vi "ALONE_3AXIS_V_AMI_DESIM.vi"(6 "Refresco(s)":dbl=1.0, 8 "error in (no error)":errorcluster) -> (0 "Error Out":errorcluster, 7 "Enable":bool=TRUE)   [LabVIEW 2017]
uses:
  cRIO_ZNB_AMI_GLOBALES.vi
  AMI MAGNET/AMI 430_Hardware_Module.ctl
  AMI MAGNET/commsControl.ctl
  AMI MAGNET/magneticField.ctl
  AMI MAGNET/Status AMI.ctl
  ALONE_3AXIS_AMI.ctl
panel:
  in  "rampingMode Z 2":u16(ring)=1 items=["RAMP", "PAUSE", "MANUAL UP", "MANUAL DOWN", "ZERO"]
  in  "x":dbl min=-0.5 max=0.5 step=0.001 format="%.2f"
  in  "y":dbl min=-0.5 max=0.5 step=0.001 format="%.2f"
  in  "Vector":bool
  in  "Demag X":bool
  out "Remote DEMAG Z":bool
  out "Remote DEMAG X":bool
  out "Remote DEMAG Y":bool
  in  "Demag Y":bool
  in  "Demag Z":bool
  out "String":string="Estado"
  out "Command":T1
  out "Remote RAMP Z":bool
  out "Remote SET X":bool
  out "Remote SET Y":bool
  out "Remote RAMP X":bool
  out "Remote RAMP Y":bool
  out "Remote SET Z":bool
  in  "rampingMode X":u16(ring)=1 items=["RAMP", "PAUSE", "MANUAL UP", "MANUAL DOWN", "ZERO"]
  in  "rampingMode Y":u16(ring)=1 items=["RAMP", "PAUSE", "MANUAL UP", "MANUAL DOWN", "ZERO"]
  in  "rampingMode Z":u16(ring)=1 items=["RAMP", "PAUSE", "MANUAL UP", "MANUAL DOWN", "ZERO"]
  in  "RAMP Z":bool
  in  "SET X":bool
  out "X ramping":bool caption="Stable"
  out "X state":T2=1 items=["Unknown", "RAMPING to target field/current", "HOLDING at the target field/current", "PAUSED", "Ramping in MANUAL UP mode", "Ramping in MANUAL DOWN mode", "ZEROING CURRENT (in progress)", "Quench detected", "At ZERO current", "Heating persistent switch", "Cooling persistent switch", "External Rampdown active"]
  in  "Target X(T)":dbl min=-0.5 max=0.5 step=0.001 format="%.2f"
  in  "Rate X(T/min)":dbl=0.1 min=0.0 max=0.1 step=0.001 format="%.2f"
  out "X field (T)":dbl format="%.2f"
  in  "SET Y":bool
  out "Y ramping":bool caption="Stable"
  out "Y state":T2=1 items=["Unknown", "RAMPING to target field/current", "HOLDING at the target field/current", "PAUSED", "Ramping in MANUAL UP mode", "Ramping in MANUAL DOWN mode", "ZEROING CURRENT (in progress)", "Quench detected", "At ZERO current", "Heating persistent switch", "Cooling persistent switch", "External Rampdown active"]
  in  "Target Y(T)":dbl min=-0.5 max=0.5 step=0.001 format="%.2f"
  in  "Rate Y(T/min)":dbl=0.1 min=0.0 max=0.1 step=0.001 format="%.2f"
  out "Y field (T)":dbl format="%.2f"
  in  "RAMP X":bool
  in  "RAMP Y":bool
  in  "Settings Z":T3={"magneticFieldUnits"=1, "rampRateUnits"=1, "rampRate"=0.0, "targetField"=0.0, "rampingMode"=1} {"rampingMode" items=["RAMP", "PAUSE", "MANUAL UP", "MANUAL DOWN", "ZERO"]; "targetField" format="%.3f"; "rampRate" format="%.3f"; "rampRateUnits" items=["Per SECOND", "Per MINUTE"]; "magneticFieldUnits" items=["KGauss", "Tesla"]}
  in  "Settings Y":T3={"magneticFieldUnits"=1, "rampRateUnits"=1, "rampRate"=0.0, "targetField"=0.0, "rampingMode"=1} {"rampingMode" items=["RAMP", "PAUSE", "MANUAL UP", "MANUAL DOWN", "ZERO"]; "targetField" format="%.3f"; "rampRate" format="%.3f"; "rampRateUnits" items=["Per SECOND", "Per MINUTE"]; "magneticFieldUnits" items=["KGauss", "Tesla"]}
  in  "Settings X":T3={"magneticFieldUnits"=1, "rampRateUnits"=1, "rampRate"=0.0, "targetField"=0.0, "rampingMode"=1} {"rampingMode" items=["RAMP", "PAUSE", "MANUAL UP", "MANUAL DOWN", "ZERO"]; "targetField" format="%.3f"; "rampRate" format="%.3f"; "rampRateUnits" items=["Per SECOND", "Per MINUTE"]; "magneticFieldUnits" items=["KGauss", "Tesla"]}
  out "Waveform Chart":T4(graph)
  in  "SET Z":bool
  out "Z ramping":bool caption="Stable"
  out "Z state":T2=1 items=["Unknown", "RAMPING to target field/current", "HOLDING at the target field/current", "PAUSED", "Ramping in MANUAL UP mode", "Ramping in MANUAL DOWN mode", "ZEROING CURRENT (in progress)", "Quench detected", "At ZERO current", "Heating persistent switch", "Cooling persistent switch", "External Rampdown active"]
  out "Ciclo":i32
  in  "Target Z(T)":dbl min=-2.0 max=2.0 step=0.001 format="%.2f"
  in  "Rate Z(T/min)":dbl=0.1 min=0.0 max=0.1 step=0.001 format="%.2f"
  out "Z field (T)":dbl format="%.2f"
  out "ERROR":bool
  out "Date":string caption="asd"
  out "Time":string caption="asd"
  in  "Refresh":bool
  in  "stop":bool
  # "X axis"
  # "Z axis"
  # "STATUS"
  # "Y axis"
  # "STATUS"
  # "STATUS"
  # "SETTINGS"
  # "SETTINGS"
  # "SETTINGS"
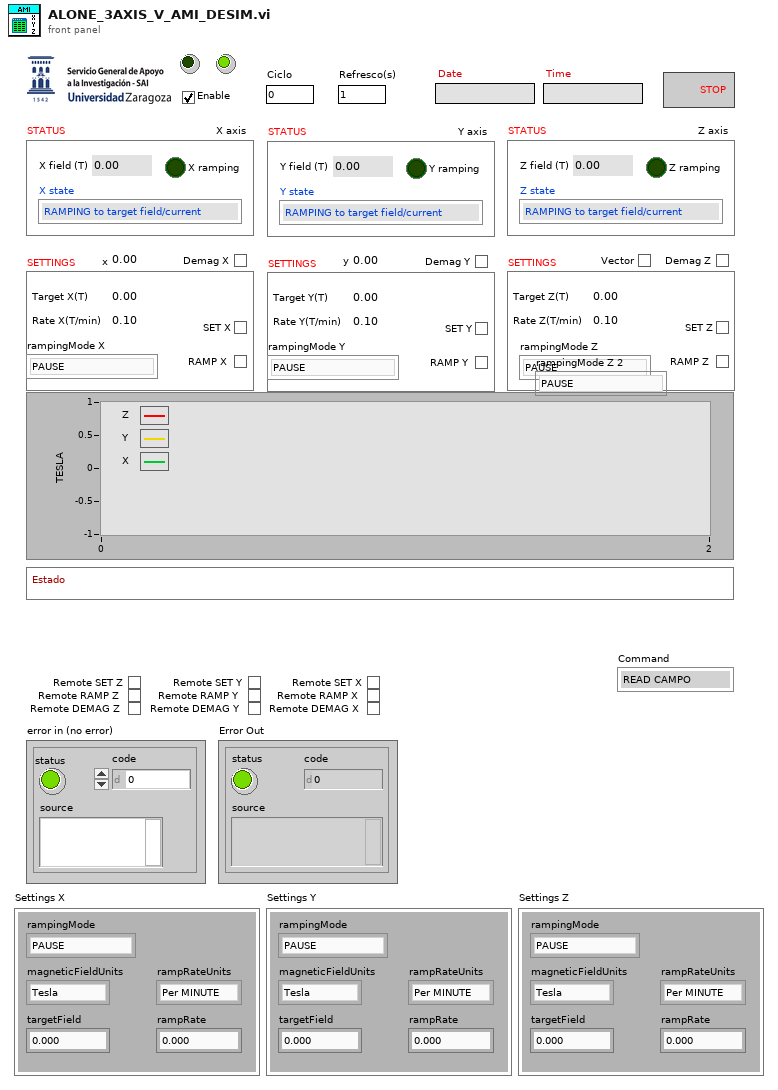
[diagram p1: front panel]
types:
  T1 = typedef "ALONE_3AXIS_AMI.ctl" = enum16{"READ CAMPO", "SET X", "SET Y", "SET Z", "RAMP X", "RAMP Y", "RAMP Z", "DESIMANAR X", "DESIMANAR Y", "DESIMANAR Z", "DESIMANAR X_RUN", "DESIMANAR Y_RUN", "DESIMANAR Z_RUN"}
  T2 = typedef "Status AMI.ctl" = u16
  T3 = typedef "magneticField.ctl" = cluster{"magneticFieldUnits":u16, "rampRateUnits":u16, "rampRate":dbl, "targetField":dbl, "rampingMode":u16}
  T4 = cluster{"magneticField":dbl, "magneticField":dbl, "magneticField":dbl}
  T5 = typedef "AMI 430_Hardware_Module.ctl" = enum16{"INICIALIZAR", "SET UNIDADES CAMPO", "SET UNIDADES RAMPA", "SET CAMPO", "SET  RAMPA", "SET RAMPING MODE", "READ CAMPO", "STATUS", "SHUTDOWN"}
  T6 = typedef "ALONE_3AXIS_AMI.ctl" = enum16{"READ CAMPO", "SET X", "SET Y", "SET Z", "RAMP X", "RAMP Y", "RAMP Z", "VECTOR Z", "DESIMANAR X", "DESIMANAR Y", "DESIMANAR Z", "DESIMANAR X_RUN", "DESIMANAR Y_RUN", "DESIMANAR Z_RUN"}
  T7 = typedef "commsControl.ctl" = cluster{"connection ID":refnum<k5>, "IP":string, "Active Comm Interface":u16, "Serial Port":refnum<visa-resource-name>, "Programmer Type":u16, "connection ID":refnum<k5>, "output cluster":cluster{"GPIB address":i16, "GPIB bus":i16}}
  T8 = cluster{"Z field (T)":dbl, "Y field (T)":dbl, "magneticField":dbl}
  T9 = cluster{"Z field (T)":dbl, "magneticField":dbl, "X field (T)":dbl}
  T10 = cluster{"magneticField":dbl, "Y field (T)":dbl, "X field (T)":dbl}
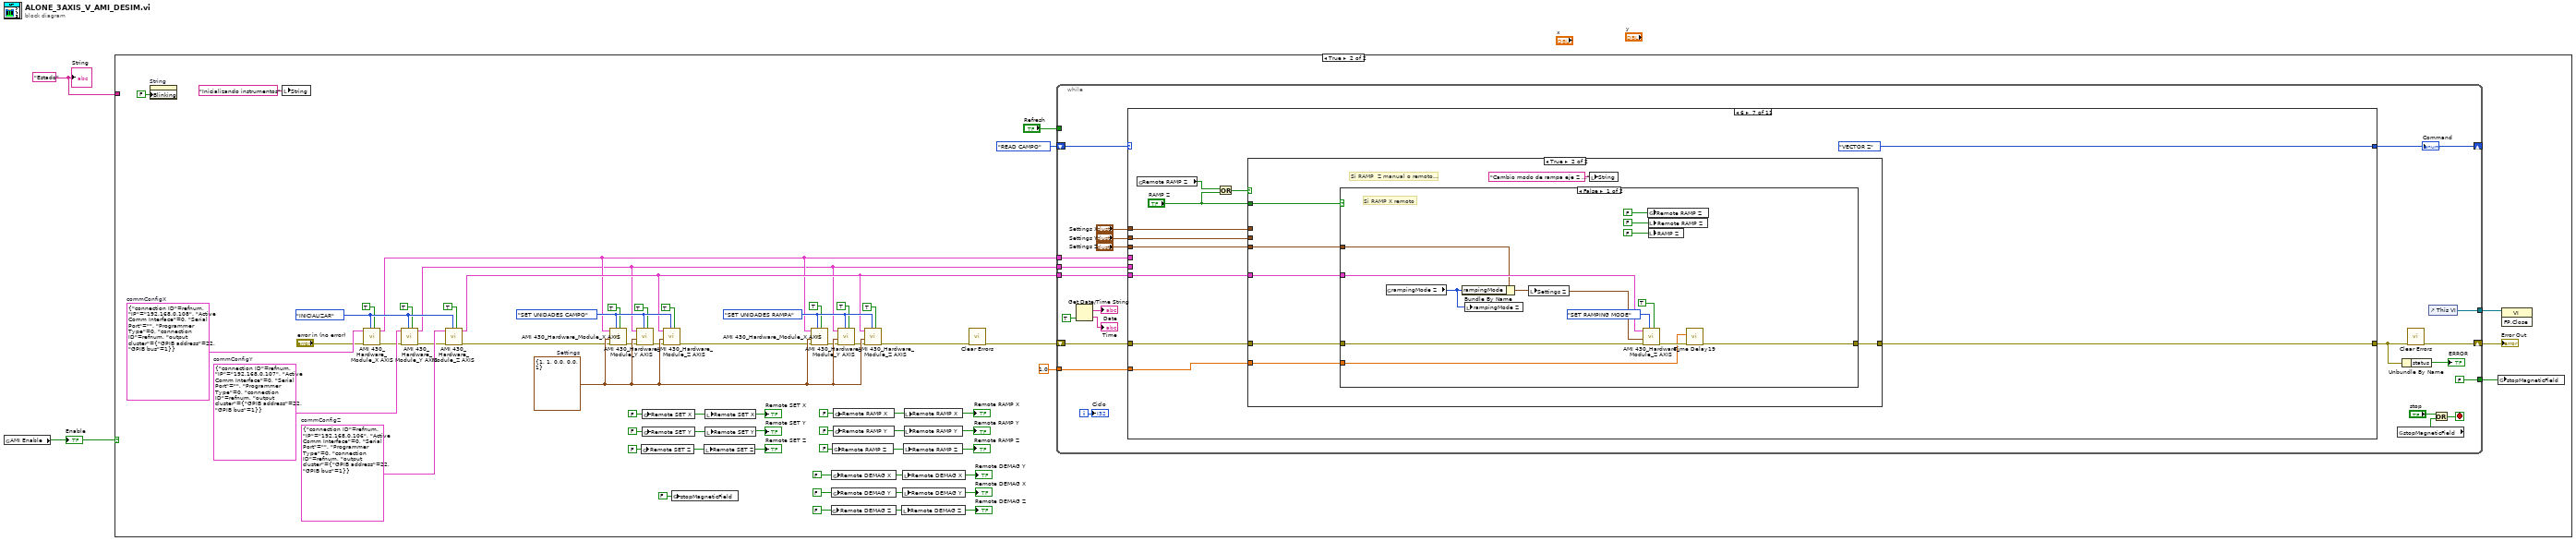
[diagram p0: block diagram]
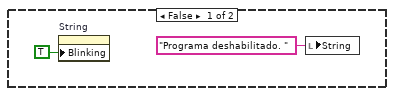
[diagram p2: hidden frame]
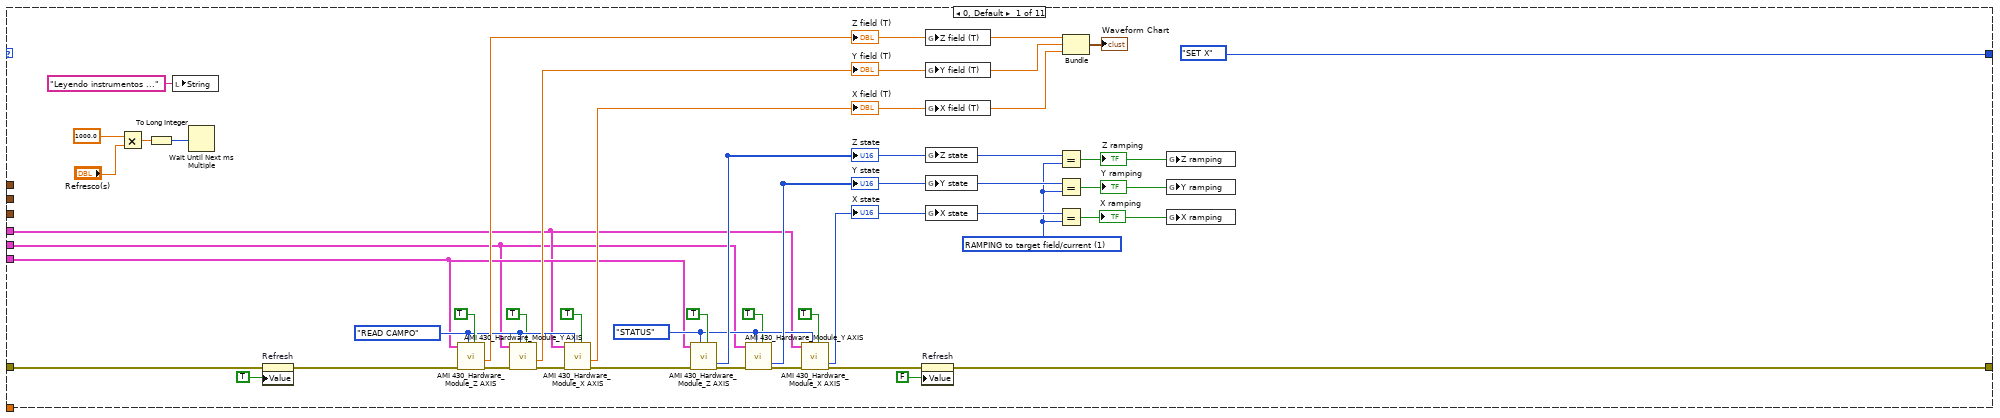
[diagram p3: hidden frame]
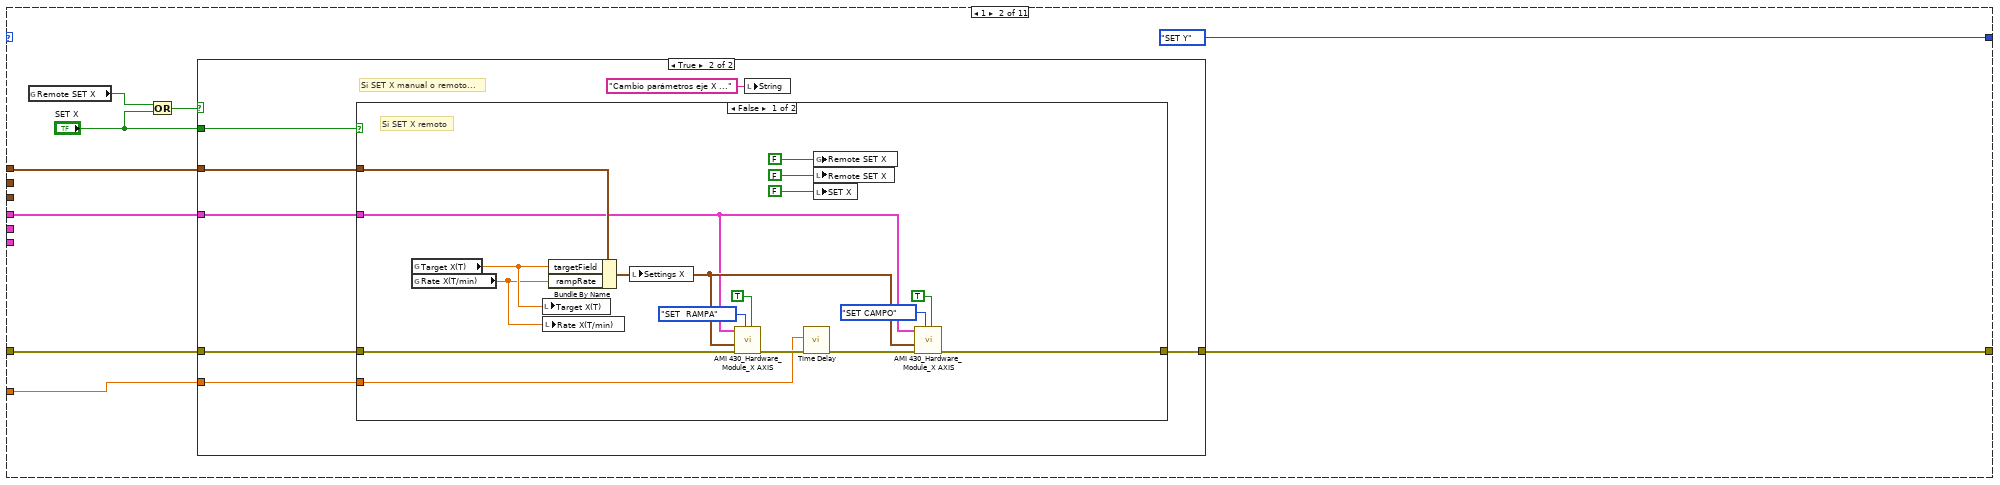
[diagram p4: hidden frame]
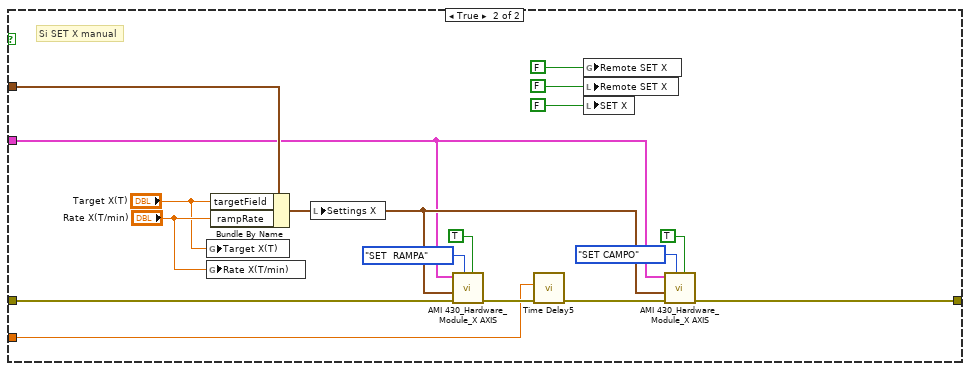
[diagram p6: hidden frame]
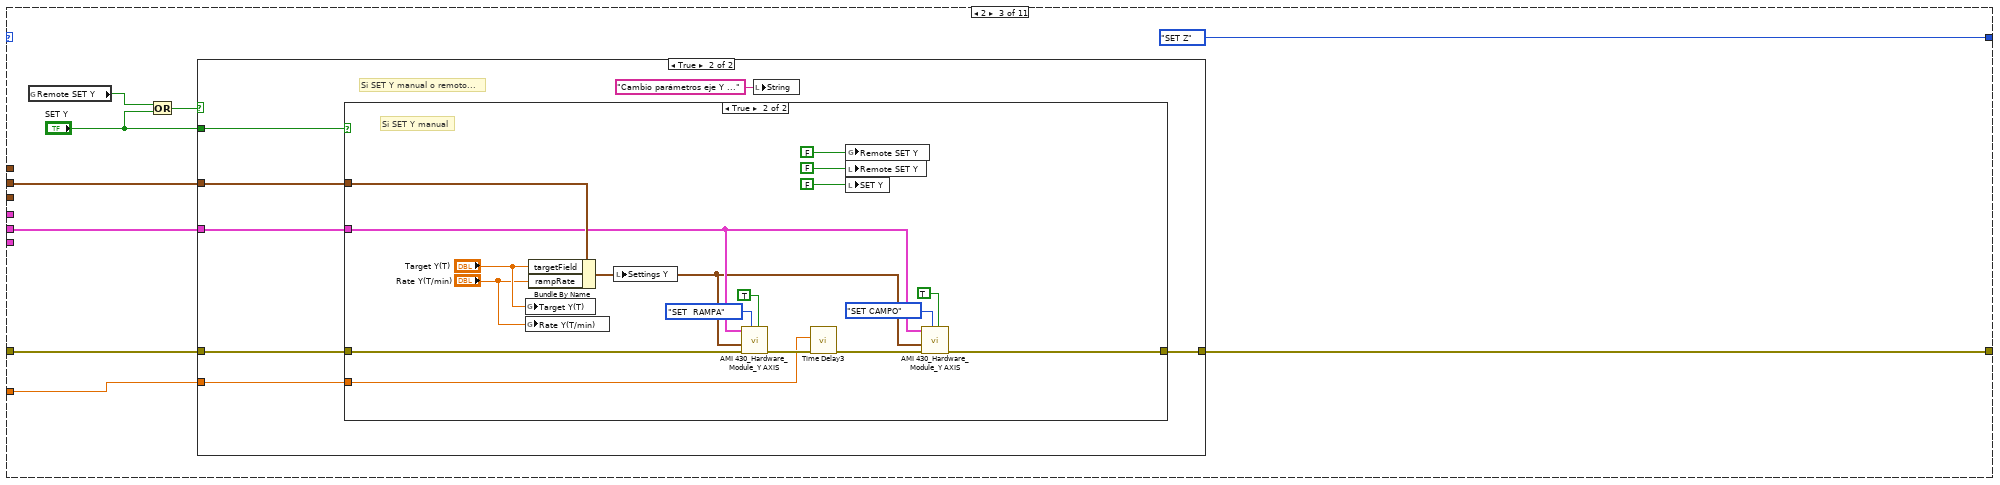
[diagram p7: hidden frame]
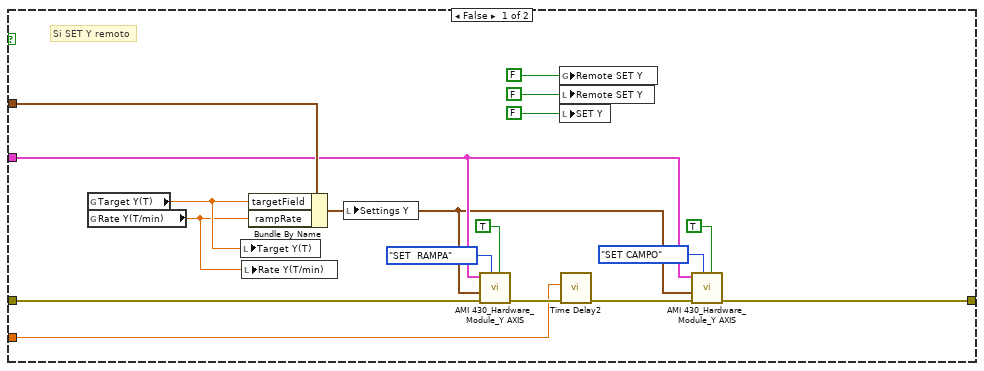
[diagram p9: hidden frame]
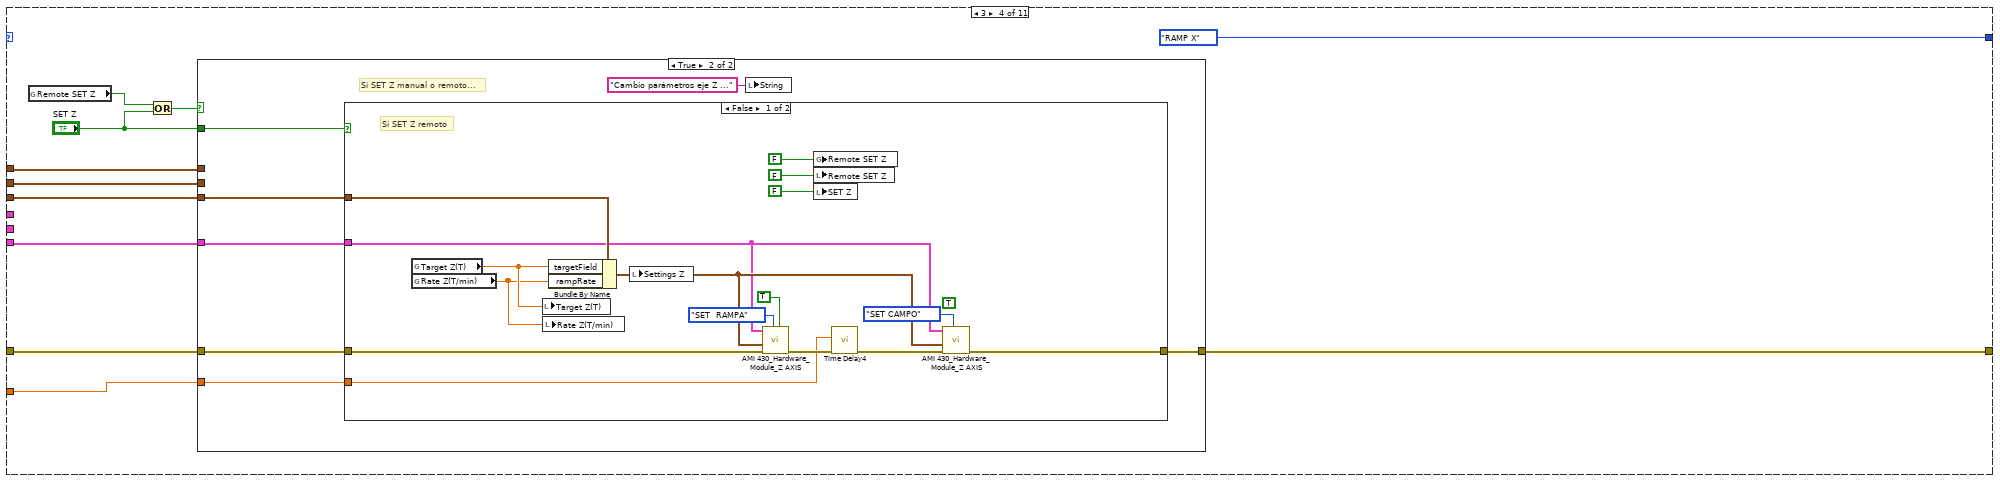
[diagram p10: hidden frame]
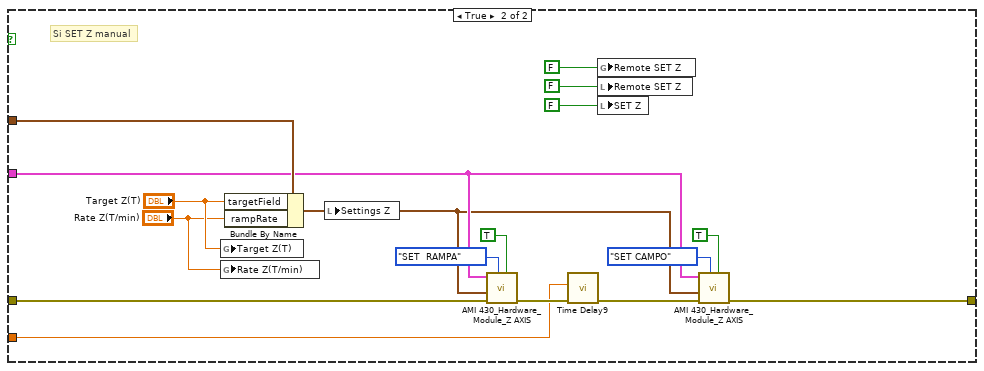
[diagram p12: hidden frame]
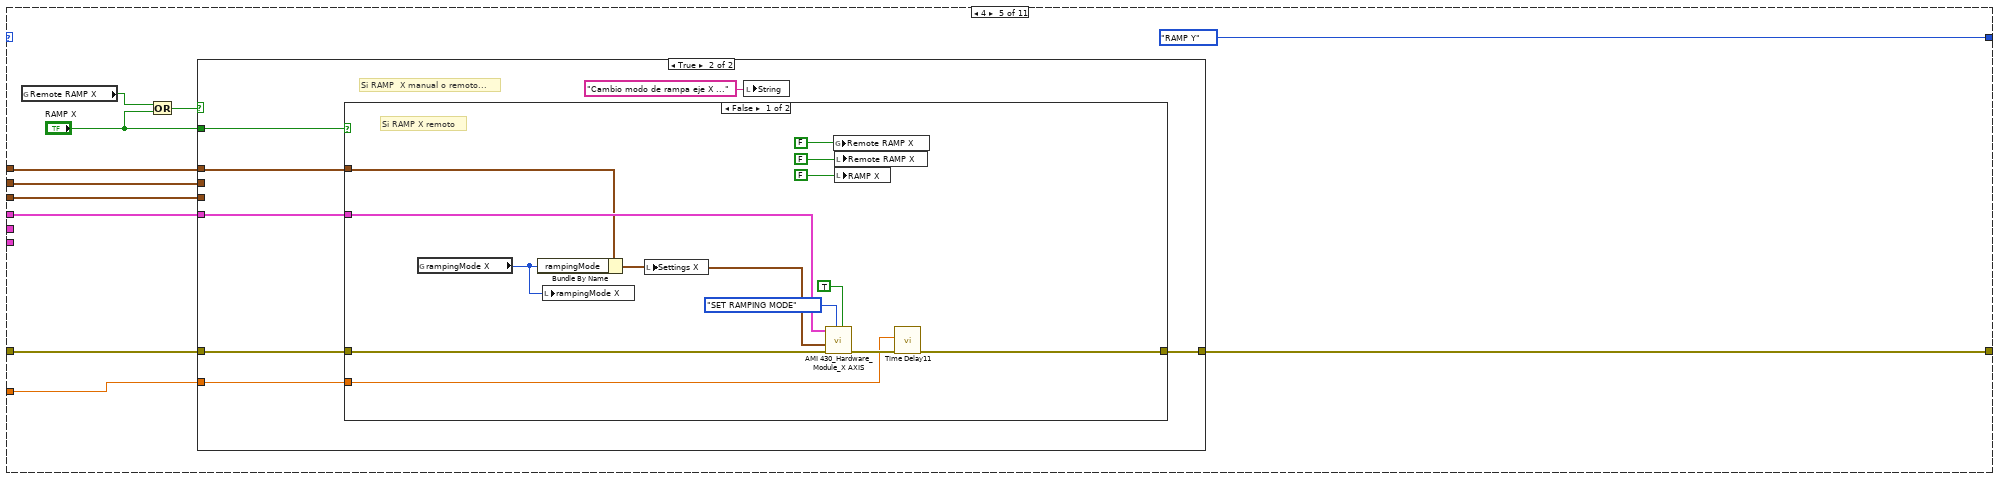
[diagram p13: hidden frame]
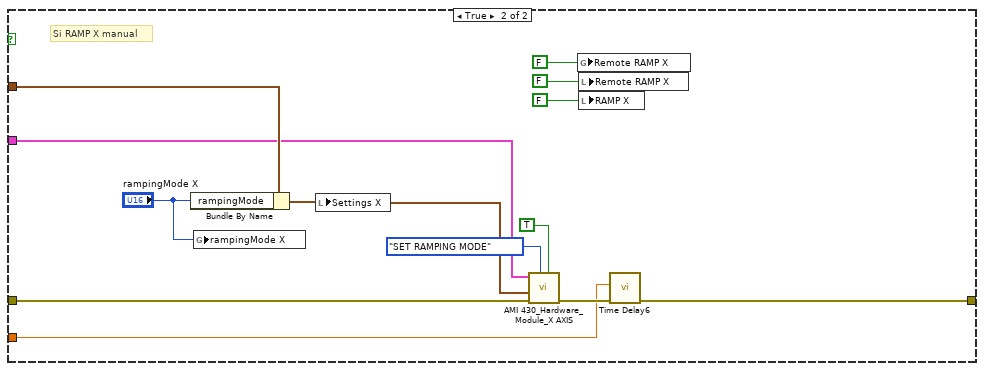
[diagram p15: hidden frame]
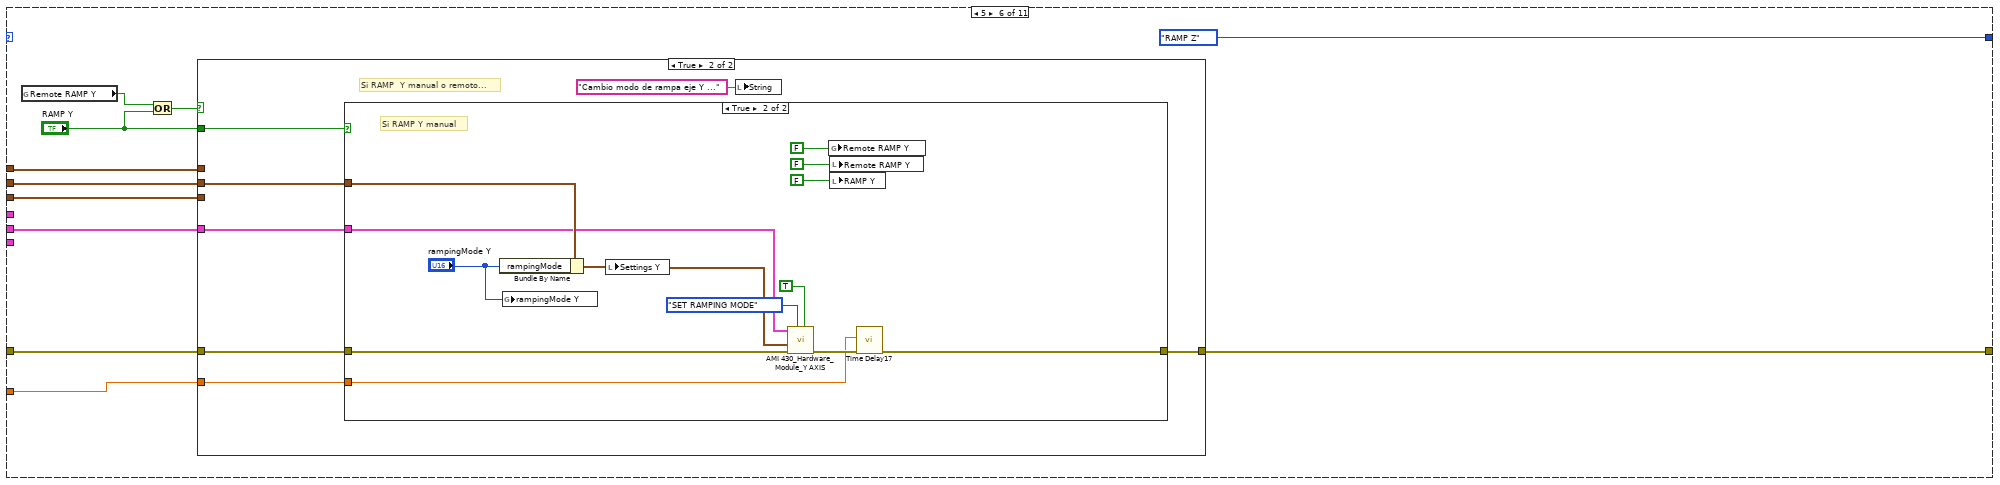
[diagram p16: hidden frame]
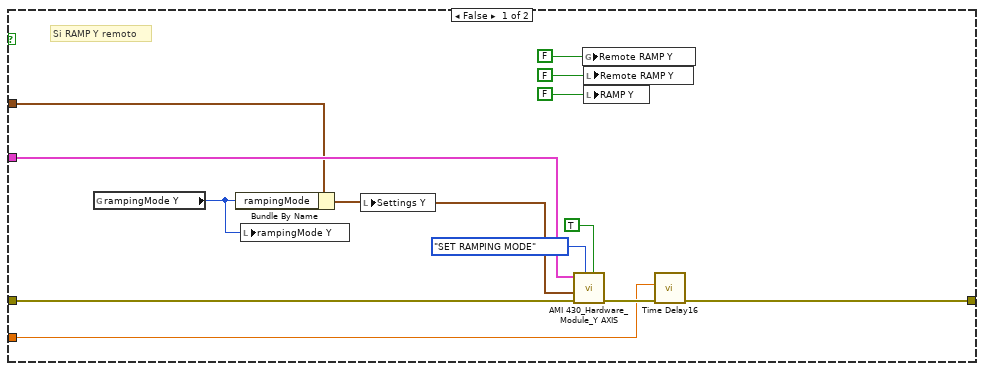
[diagram p18: hidden frame]
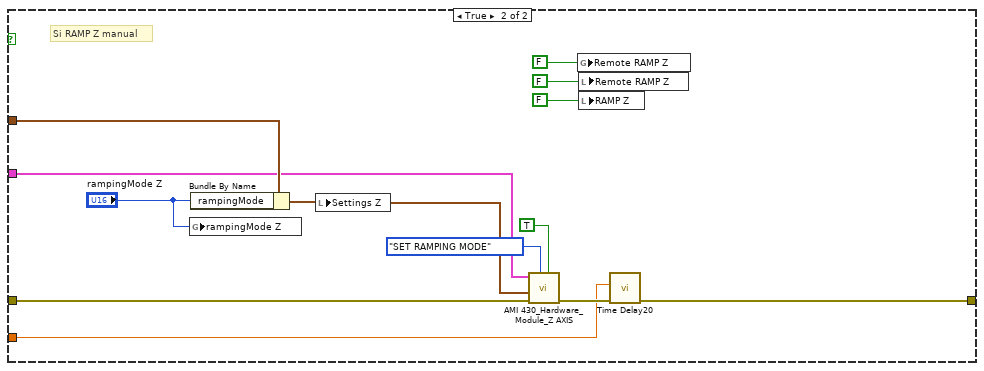
[diagram p20: hidden frame]
diagram:
  w1 = "Estado" ("String")
  n1 = global read "cRIO_ZNB_AMI_GLOBALES.vi" "AMI Enable"() -> (w2:bool)
  "Enable" <- w2
  n2 = case shown="True" w2 {
    tunnel: w1 -> [_ _]
    frame False {
      n3 = property on="String" class="Str"("Blinking"=TRUE) -> ()  [unwired: 2 in, 2 out]
      n4 = local write "String"("Programa deshabilitado. " ("String")) -> ()
    }
    frame True {
      w5 = FALSE ("Remote RAMP Z")
      w6 = FALSE ("Remote RAMP Y")
      w7 = FALSE ("Remote RAMP X")
      w12 = FALSE ("Remote SET Z")
      w11 = FALSE ("Remote SET Y")
      w13 = FALSE ("Remote SET X")
      w16 = FALSE ("Remote RAMP Z")
      w15 = FALSE ("Remote RAMP Y")
      w14 = FALSE ("Remote RAMP X")
      w45 = T3 {"magneticFieldUnits"=1, "rampRateUnits"=1, "rampRate"=0.0, "targetField"=0.0, "rampingMode"=1}  # Settings
      w41 = AMI_430_Hardware_Module."SET UNIDADES RAMPA" ("Command")
      w40 = AMI_430_Hardware_Module."SET UNIDADES CAMPO" ("Command")
      w48 = T7 {"connection ID"=refnum, "IP"="192.168.0.106", "Active Comm Interface"=0, "Serial Port"="", "Programmer Type"=0, "connection ID"=refnum, "output cluster"={"GPIB address"=22, "GPIB bus"=1}}  # commConfigZ
      w47 = T7 {"connection ID"=refnum, "IP"="192.168.0.107", "Active Comm Interface"=0, "Serial Port"="", "Programmer Type"=0, "connection ID"=refnum, "output cluster"={"GPIB address"=22, "GPIB bus"=1}}  # commConfigY
      w46 = T7 {"connection ID"=refnum, "IP"="192.168.0.108", "Active Comm Interface"=0, "Serial Port"="", "Programmer Type"=0, "connection ID"=refnum, "output cluster"={"GPIB address"=22, "GPIB bus"=1}}  # commConfigX
      w49 = AMI_430_Hardware_Module."INICIALIZAR" ("Command")
      n5 = property on="String" class="Str"("Blinking"=FALSE) -> ()  [unwired: 2 in, 2 out]
      n6 = local write "String"("Inicializando instrumentos" ("String")) -> ()
      n7 = call "AMI 430_Hardware_Module_X AXIS.vi"("Enable"=TRUE, "Command"=w49, "error in (no error)"="error in (no error)", "Comm Config In"=w46) -> ("error out"=w36:errorcluster, "Comm Config Out"=w20:T7)  [unwired: 3 in, 3 out]
      n8 = call "AMI 430_Hardware_Module_Y AXIS.vi"("Enable"=TRUE, "Command"=w49, "error in (no error)"=w36, "Comm Config In"=w47) -> ("error out"=w35:errorcluster, "Comm Config Out"=w19:T7)  [unwired: 3 in, 3 out]
      n9 = call "AMI 430_Hardware_Module_Z AXIS.vi"("Enable"=TRUE, "Command"=w49, "error in (no error)"=w35, "Comm Config In"=w48) -> ("error out"=w39:errorcluster, "Comm Config Out"=w21:T7)  [unwired: 3 in, 3 out]
      n10 = call "AMI 430_Hardware_Module_X AXIS.vi"("Enable"=TRUE, "Command"=w40, "error in (no error)"=w39, "Settings"=w45, "Comm Config In"=w20) -> ("error out"=w37:errorcluster)  [unwired: 2 in, 4 out]
      n11 = call "AMI 430_Hardware_Module_Y AXIS.vi"("Enable"=TRUE, "Command"=w40, "error in (no error)"=w37, "Settings"=w45, "Comm Config In"=w19) -> ("error out"=w38:errorcluster)  [unwired: 2 in, 4 out]
      n12 = global write "cRIO_ZNB_AMI_GLOBALES.vi" "Remote SET Z"(w12) -> ()
      n13 = global write "cRIO_ZNB_AMI_GLOBALES.vi" "Remote SET X"(w13) -> ()
      n14 = global write "cRIO_ZNB_AMI_GLOBALES.vi" "Remote SET Y"(w11) -> ()
      n15 = call "AMI 430_Hardware_Module_Z AXIS.vi"("Enable"=TRUE, "Command"=w40, "error in (no error)"=w38, "Settings"=w45, "Comm Config In"=w21) -> ("error out"=w44:errorcluster)  [unwired: 2 in, 4 out]
      n16 = global write "cRIO_ZNB_AMI_GLOBALES.vi" "stopMagneticField"(FALSE ("stopMagneticField")) -> ()
      n17 = local write "Remote SET Z"(w12) -> ()
      n18 = local write "Remote SET X"(w13) -> ()
      n19 = local write "Remote SET Y"(w11) -> ()
      n20 = call "AMI 430_Hardware_Module_X AXIS.vi"("Enable"=TRUE, "Command"=w41, "error in (no error)"=w44, "Settings"=w45, "Comm Config In"=w20) -> ("error out"=w42:errorcluster)  [unwired: 2 in, 4 out]
      n21 = global write "cRIO_ZNB_AMI_GLOBALES.vi" "Remote DEMAG Z"(w5) -> ()
      n22 = global write "cRIO_ZNB_AMI_GLOBALES.vi" "Remote DEMAG X"(w7) -> ()
      n23 = global write "cRIO_ZNB_AMI_GLOBALES.vi" "Remote DEMAG Y"(w6) -> ()
      n24 = global write "cRIO_ZNB_AMI_GLOBALES.vi" "Remote RAMP Z"(w16) -> ()
      n25 = global write "cRIO_ZNB_AMI_GLOBALES.vi" "Remote RAMP X"(w14) -> ()
      n26 = global write "cRIO_ZNB_AMI_GLOBALES.vi" "Remote RAMP Y"(w15) -> ()
      n27 = call "AMI 430_Hardware_Module_Y AXIS.vi"("Enable"=TRUE, "Command"=w41, "error in (no error)"=w42, "Settings"=w45, "Comm Config In"=w19) -> ("error out"=w43:errorcluster)  [unwired: 2 in, 4 out]
      n28 = call "AMI 430_Hardware_Module_Z AXIS.vi"("Enable"=TRUE, "Command"=w41, "error in (no error)"=w43, "Settings"=w45, "Comm Config In"=w21) -> ("error out"=w34:errorcluster)  [unwired: 2 in, 4 out]
      n29 = local write "Remote DEMAG Z"(w5) -> ()
      n30 = local write "Remote DEMAG X"(w7) -> ()
      n31 = local write "Remote DEMAG Y"(w6) -> ()
      n32 = local write "Remote RAMP Z"(w16) -> ()
      n33 = local write "Remote RAMP X"(w14) -> ()
      n34 = local write "Remote RAMP Y"(w15) -> ()
      n35 = call <vilib>:"Clear Errors.vi"("error in (no error)"=w34) -> ("error out"=w18:errorcluster)  [unwired: 5 in, 1 out]
      n36 = while {
        shift-right: [w65] -> w50
        shift-left: w18 -> [w58]
        tunnel: [FALSE ("stop")] -> w51
        tunnel: [w68] -> w52
        tunnel: "Refresh" -> [_]
        tunnel: w19 -> [w59]
        tunnel: w21 -> [w60]
        tunnel: w20 -> [w61]
        shift-right: [w54] -> _
        shift-left: ALONE_3AXIS_AMI."READ CAMPO" ("Command") -> [w63]
        tunnel: 1.0 ("Delay Time (s)") -> [w53]
        i -> [w64]
        stop <- w72 stop-if-true
        n37 = Get Date/Time String(want seconds? (F)=TRUE) -> (date string=→"Date":string, time string=→"Time":string)  [unwired: 2 in]
        n38 = case shown="6" w63 {
          tunnel: w58 -> [w78 w121 w173 w225 w277 w322 w367 w412 w457 w540 w624]
          tunnel: w61 -> [w88 w117 _ _ w268 _ _ _ w449 _ _]
          tunnel: w59 -> [w87 _ w165 _ _ w314 _ _ _ w531 _]
          tunnel: w60 -> [w89 _ _ w216 _ _ w358 w404 _ _ w615]
          tunnel: [w75 w120 w172 w224 w276 w321 w366 w411 w456 w539 w623] -> w62
          tunnel: "Settings Y" -> [_ _ w166 w217 w270 w315 w360 w405 w450 w533 w617]
          tunnel: "Settings Z" -> [_ _ _ w218 w271 w316 w361 w406 w451 w534 w618]
          tunnel: "Settings X" -> [_ w122 _ w226 w278 w323 w368 w413 w458 w541 w625]
          tunnel: [ALONE_3AXIS_AMI."SET X" ("Command") ALONE_3AXIS_AMI."SET Y" ("Command") ALONE_3AXIS_AMI."SET Z" ("Command") ALONE_3AXIS_AMI."RAMP X" ("Command") ALONE_3AXIS_AMI."RAMP Y" ("Command") ALONE_3AXIS_AMI."RAMP Z" ("Command") ALONE_3AXIS_AMI."VECTOR Z" ("Command") ALONE_3AXIS_AMI."DESIMANAR X" ("Command") ALONE_3AXIS_AMI."DESIMANAR Y" ("Command") ALONE_3AXIS_AMI."DESIMANAR Z" ("Command") ALONE_3AXIS_AMI."READ CAMPO" ("Command")] -> w54
          tunnel: w53 -> [_ w118 w170 w222 w274 w319 w364 w409 w454 w537 w621]
          frame 0, Default {
            w98 = T2 1 items=["Unknown", "RAMPING to target field/current", "HOLDING at the target field/current", "PAUSED", "Ramping in MANUAL UP mode", "Ramping in MANUAL DOWN mode", "ZEROING CURRENT (in progress)", "Quench detected", "At ZERO current", "Heating persistent switch", "Cooling persistent switch", "External Rampdown active"] ("y")
            w96 = AMI_430_Hardware_Module."STATUS" ("Command")
            w92 = AMI_430_Hardware_Module."READ CAMPO" ("Command")
            n39 = Multiply(x=1000.0, y="Refresco(s)") -> (x*y=w83:dbl)
            n40 = To Long Integer(number=w83) -> (32bit integer=w81:i32)
            n41 = local write "String"("Leyendo instrumentos ..." ("String")) -> ()
            n42 = Wait Until Next ms Multiple(millisecond multiple=w81) -> ()  [unwired: 1 out]
            n43 = property on="Refresh" class="Bool (strict)"(error in=w78, "Value"=TRUE ("Refresh")) -> (error out=w77:errorcluster)  [unwired: 1 in, 1 out]
            n44 = call "AMI 430_Hardware_Module_Z AXIS.vi"("Enable"=TRUE, "Command"=w92, "error in (no error)"=w77, "Comm Config In"=w89) -> ("error out"=w100:errorcluster, "magneticField"=w110:dbl)  [unwired: 3 in, 3 out]
            "Z field (T)" <- w110
            n45 = call "AMI 430_Hardware_Module_Y AXIS.vi"("Enable"=TRUE, "Command"=w92, "error in (no error)"=w100, "Comm Config In"=w87) -> ("error out"=w99:errorcluster, "magneticField"=w109:dbl)  [unwired: 3 in, 3 out]
            "Y field (T)" <- w109
            n46 = call "AMI 430_Hardware_Module_X AXIS.vi"("Enable"=TRUE, "Command"=w92, "error in (no error)"=w99, "Comm Config In"=w88) -> ("error out"=w101:errorcluster, "magneticField"=w108:dbl)  [unwired: 3 in, 3 out]
            "X field (T)" <- w108
            n47 = call "AMI 430_Hardware_Module_Z AXIS.vi"("Enable"=TRUE, "Command"=w96, "error in (no error)"=w101, "Comm Config In"=w89) -> ("error out"=w103:errorcluster, "state"=w111:T2)  [unwired: 3 in, 3 out]
            "Z state" <- w111
            n48 = call "AMI 430_Hardware_Module_Y AXIS.vi"("Enable"=TRUE, "Command"=w96, "error in (no error)"=w103, "Comm Config In"=w87) -> ("error out"=w102:errorcluster, "state"=w112:T2)  [unwired: 3 in, 3 out]
            "Y state" <- w112
            n49 = call "AMI 430_Hardware_Module_X AXIS.vi"("Enable"=TRUE, "Command"=w96, "error in (no error)"=w102, "Comm Config In"=w88) -> ("error out"=w76:errorcluster, "state"=w113:T2)  [unwired: 3 in, 3 out]
            "X state" <- w113
            n50 = property on="Refresh" class="Bool (strict)"(error in=w76, "Value"=FALSE ("Refresh")) -> (error out=w75:errorcluster)  [unwired: 1 in, 1 out]
            n51 = global write "cRIO_ZNB_AMI_GLOBALES.vi" "Z field (T)"(w110) -> ()
            n52 = global write "cRIO_ZNB_AMI_GLOBALES.vi" "Y field (T)"(w109) -> ()
            n53 = global write "cRIO_ZNB_AMI_GLOBALES.vi" "X field (T)"(w108) -> ()
            n54 = global write "cRIO_ZNB_AMI_GLOBALES.vi" "Z state"(w111) -> ()
            n55 = global write "cRIO_ZNB_AMI_GLOBALES.vi" "Y state"(w112) -> ()
            n56 = global write "cRIO_ZNB_AMI_GLOBALES.vi" "X state"(w113) -> ()
            n57 = Equal?(x=w111, y=w98) -> (x = y?=w105:bool)
            "Z ramping" <- w105
            n58 = Equal?(x=w112, y=w98) -> (x = y?=w107:bool)
            "Y ramping" <- w107
            n59 = Equal?(x=w113, y=w98) -> (x = y?=w106:bool)
            "X ramping" <- w106
            n60 = Bundle("magneticField"=w110, "magneticField"=w109, "magneticField"=w108) -> (→"Waveform Chart":T4)  [unwired: 1 in]
            n61 = global write "cRIO_ZNB_AMI_GLOBALES.vi" "Z ramping"(w105) -> ()
            n62 = global write "cRIO_ZNB_AMI_GLOBALES.vi" "Y ramping"(w107) -> ()
            n63 = global write "cRIO_ZNB_AMI_GLOBALES.vi" "X ramping"(w106) -> ()
          }
          frame 1 {
            n64 = global read "cRIO_ZNB_AMI_GLOBALES.vi" "Remote SET X"() -> (w116:bool)
            n65 = Or(x=w116, y="SET X") -> (x .or. y?=w115:bool)
            n66 = case shown="True" w115 {
              tunnel: w122 -> [_ w130]
              tunnel: w121 -> [w123 w129]
              tunnel: [w123 w128] -> w120
              tunnel: w118 -> [_ w127]
              tunnel: w117 -> [_ w126]
              tunnel: "SET X" -> [_ w125]
              frame False {
              }
              frame True {
                # "Si SET X manual o remoto..."
                n67 = case shown="False" w125 {
                  tunnel: w130 -> [w140 w155]
                  tunnel: w129 -> [w139 w154]
                  tunnel: [w138 w153] -> w128
                  tunnel: w127 -> [w137 w152]
                  tunnel: w126 -> [w136 w151]
                  frame False {
                    # "Si SET X remoto"
                    n68 = global read "cRIO_ZNB_AMI_GLOBALES.vi" "Target X(T)"() -> (w135:dbl)
                    n69 = global read "cRIO_ZNB_AMI_GLOBALES.vi" "Rate X(T/min)"() -> (w134:dbl)
                    n70 = local write "Target X(T)"(w135) -> ()
                    n71 = local write "Rate X(T/min)"(w134) -> ()
                    n72 = Bundle By Name(cluster=w140, "targetField"=w135, "rampRate"=w134) -> (w147:T3)
                    n73 = local write "Settings X"(w147) -> ()
                    n74 = call "AMI 430_Hardware_Module_X AXIS.vi"("Enable"=TRUE, "Command"=AMI_430_Hardware_Module."SET  RAMPA", "error in (no error)"=w139, "Settings"=w147, "Comm Config In"=w136) -> ("error out"=w145:errorcluster)  [unwired: 2 in, 4 out]
                    n75 = call "Time Delay"("error in (no error)"=w145, "Delay Time (s)"=w137) -> ("error out"=w146:errorcluster)  [unwired: 9 in]
                    n76 = global write "cRIO_ZNB_AMI_GLOBALES.vi" "Remote SET X"(FALSE ("Remote SET X")) -> ()
                    n77 = local write "Remote SET X"(FALSE ("Remote SET X")) -> ()
                    n78 = local write "SET X"(FALSE ("Remote SET X")) -> ()
                    n79 = call "AMI 430_Hardware_Module_X AXIS.vi"("Enable"=TRUE, "Command"=AMI_430_Hardware_Module."SET CAMPO", "error in (no error)"=w146, "Settings"=w147, "Comm Config In"=w136) -> ("error out"=w138:errorcluster)  [unwired: 2 in, 4 out]
                  }
                  frame True {
                    # "Si SET X manual"
                    n80 = global write "cRIO_ZNB_AMI_GLOBALES.vi" "Target X(T)"("Target X(T)") -> ()
                    n81 = global write "cRIO_ZNB_AMI_GLOBALES.vi" "Rate X(T/min)"("Rate X(T/min)") -> ()
                    n82 = Bundle By Name(cluster=w155, "targetField"="Target X(T)", "rampRate"="Rate X(T/min)") -> (w162:T3)
                    n83 = local write "Settings X"(w162) -> ()
                    n84 = call "AMI 430_Hardware_Module_X AXIS.vi"("Enable"=TRUE, "Command"=AMI_430_Hardware_Module."SET  RAMPA", "error in (no error)"=w154, "Settings"=w162, "Comm Config In"=w151) -> ("error out"=w160:errorcluster)  [unwired: 2 in, 4 out]
                    n85 = call "Time Delay5"("error in (no error)"=w160, "Delay Time (s)"=w152) -> ("error out"=w161:errorcluster)  [unwired: 9 in]
                    n86 = global write "cRIO_ZNB_AMI_GLOBALES.vi" "Remote SET X"(FALSE ("Remote SET X")) -> ()
                    n87 = local write "Remote SET X"(FALSE ("Remote SET X")) -> ()
                    n88 = local write "SET X"(FALSE ("Remote SET X")) -> ()
                    n89 = call "AMI 430_Hardware_Module_X AXIS.vi"("Enable"=TRUE, "Command"=AMI_430_Hardware_Module."SET CAMPO", "error in (no error)"=w161, "Settings"=w162, "Comm Config In"=w151) -> ("error out"=w153:errorcluster)  [unwired: 2 in, 4 out]
                  }
                }
                n90 = local write "String"("Cambio parámetros eje X ..." ("String")) -> ()
              }
            }
          }
          frame 2 {
            n91 = global read "cRIO_ZNB_AMI_GLOBALES.vi" "Remote SET Y"() -> (w169:bool)
            n92 = Or(x=w169, y="SET Y") -> (x .or. y?=w168:bool)
            n93 = case shown="True" w168 {
              tunnel: w166 -> [_ w181]
              tunnel: w173 -> [w174 w180]
              tunnel: [w174 w179] -> w172
              tunnel: w170 -> [_ w178]
              tunnel: w165 -> [_ w177]
              tunnel: "SET Y" -> [_ w176]
              frame False {
              }
              frame True {
                # "Si SET Y manual o remoto..."
                n94 = case shown="True" w176 {
                  tunnel: w181 -> [w198 w215]
                  tunnel: w180 -> [w184 w205]
                  tunnel: [w182 w204] -> w179
                  tunnel: w178 -> [w183 w203]
                  tunnel: w177 -> [w186 w202]
                  frame False {
                    # "Si SET Y remoto"
                    n95 = global read "cRIO_ZNB_AMI_GLOBALES.vi" "Target Y(T)"() -> (w197:dbl)
                    n96 = global read "cRIO_ZNB_AMI_GLOBALES.vi" "Rate Y(T/min)"() -> (w196:dbl)
                    n97 = local write "Target Y(T)"(w197) -> ()
                    n98 = local write "Rate Y(T/min)"(w196) -> ()
                    n99 = Bundle By Name(cluster=w198, "targetField"=w197, "rampRate"=w196) -> (w185:T3)
                    n100 = local write "Settings Y"(w185) -> ()
                    n101 = call "AMI 430_Hardware_Module_Y AXIS.vi"("Enable"=TRUE, "Command"=AMI_430_Hardware_Module."SET  RAMPA", "error in (no error)"=w184, "Settings"=w185, "Comm Config In"=w186) -> ("error out"=w192:errorcluster)  [unwired: 2 in, 4 out]
                    n102 = global write "cRIO_ZNB_AMI_GLOBALES.vi" "Remote SET Y"(FALSE ("Remote SET X")) -> ()
                    n103 = local write "Remote SET Y"(FALSE ("Remote SET X")) -> ()
                    n104 = local write "SET Y"(FALSE ("Remote SET X")) -> ()
                    n105 = call "Time Delay2"("error in (no error)"=w192, "Delay Time (s)"=w183) -> ("error out"=w190:errorcluster)  [unwired: 9 in]
                    n106 = call "AMI 430_Hardware_Module_Y AXIS.vi"("Enable"=TRUE, "Command"=AMI_430_Hardware_Module."SET CAMPO", "error in (no error)"=w190, "Settings"=w185, "Comm Config In"=w186) -> ("error out"=w182:errorcluster)  [unwired: 2 in, 4 out]
                  }
                  frame True {
                    # "Si SET Y manual"
                    n107 = global write "cRIO_ZNB_AMI_GLOBALES.vi" "Target Y(T)"("Target Y(T)") -> ()
                    n108 = global write "cRIO_ZNB_AMI_GLOBALES.vi" "Rate Y(T/min)"("Rate Y(T/min)") -> ()
                    n109 = Bundle By Name(cluster=w215, "targetField"="Target Y(T)", "rampRate"="Rate Y(T/min)") -> (w201:T3)
                    n110 = local write "Settings Y"(w201) -> ()
                    n111 = call "AMI 430_Hardware_Module_Y AXIS.vi"("Enable"=TRUE, "Command"=AMI_430_Hardware_Module."SET  RAMPA", "error in (no error)"=w205, "Settings"=w201, "Comm Config In"=w202) -> ("error out"=w211:errorcluster)  [unwired: 2 in, 4 out]
                    n112 = call "Time Delay3"("error in (no error)"=w211, "Delay Time (s)"=w203) -> ("error out"=w209:errorcluster)  [unwired: 9 in]
                    n113 = global write "cRIO_ZNB_AMI_GLOBALES.vi" "Remote SET Y"(FALSE ("Remote SET X")) -> ()
                    n114 = local write "Remote SET Y"(FALSE ("Remote SET X")) -> ()
                    n115 = local write "SET Y"(FALSE ("Remote SET X")) -> ()
                    n116 = call "AMI 430_Hardware_Module_Y AXIS.vi"("Enable"=TRUE, "Command"=AMI_430_Hardware_Module."SET CAMPO", "error in (no error)"=w209, "Settings"=w201, "Comm Config In"=w202) -> ("error out"=w204:errorcluster)  [unwired: 2 in, 4 out]
                  }
                }
                n117 = local write "String"("Cambio parámetros eje Y ..." ("String")) -> ()
              }
            }
          }
          frame 3 {
            n118 = global read "cRIO_ZNB_AMI_GLOBALES.vi" "Remote SET Z"() -> (w221:bool)
            n119 = Or(x=w221, y="SET Z") -> (x .or. y?=w220:bool)
            n120 = case shown="True" w220 {
              tunnel: w226 -> [_ _]
              tunnel: w225 -> [w227 w234]
              tunnel: [w227 w233] -> w224
              tunnel: w222 -> [_ w232]
              tunnel: w216 -> [_ w231]
              tunnel: "SET Z" -> [_ w230]
              tunnel: w218 -> [_ w229]
              tunnel: w217 -> [_ _]
              frame False {
              }
              frame True {
                # "Si SET Z manual o remoto..."
                n121 = case shown="False" w230 {
                  tunnel: w229 -> [w250 w267]
                  tunnel: w234 -> [w238 w257]
                  tunnel: [w237 w256] -> w233
                  tunnel: w232 -> [w239 w253]
                  tunnel: w231 -> [w235 w255]
                  frame False {
                    (unwired) TRUE ("Enable")
                    # "Si SET Z remoto"
                    n122 = global read "cRIO_ZNB_AMI_GLOBALES.vi" "Target Z(T)"() -> (w249:dbl)
                    n123 = global read "cRIO_ZNB_AMI_GLOBALES.vi" "Rate Z(T/min)"() -> (w248:dbl)
                    n124 = local write "Target Z(T)"(w249) -> ()
                    n125 = local write "Rate Z(T/min)"(w248) -> ()
                    n126 = Bundle By Name(cluster=w250, "targetField"=w249, "rampRate"=w248) -> (w236:T3)
                    n127 = local write "Settings Z"(w236) -> ()
                    n128 = call "AMI 430_Hardware_Module_Z AXIS.vi"("Enable"=TRUE, "Command"=AMI_430_Hardware_Module."SET  RAMPA", "error in (no error)"=w238, "Settings"=w236, "Comm Config In"=w235) -> ("error out"=w241:errorcluster)  [unwired: 2 in, 4 out]
                    n129 = global write "cRIO_ZNB_AMI_GLOBALES.vi" "Remote SET Z"(FALSE ("Remote SET X")) -> ()
                    n130 = local write "Remote SET Z"(FALSE ("Remote SET X")) -> ()
                    n131 = local write "SET Z"(FALSE ("Remote SET X")) -> ()
                    n132 = call "Time Delay4"("error in (no error)"=w241, "Delay Time (s)"=w239) -> ("error out"=w240:errorcluster)  [unwired: 9 in]
                    n133 = call "AMI 430_Hardware_Module_Z AXIS.vi"("Command"=AMI_430_Hardware_Module."SET CAMPO", "error in (no error)"=w240, "Settings"=w236, "Comm Config In"=w235) -> ("error out"=w237:errorcluster)  [unwired: 3 in, 4 out]
                  }
                  frame True {
                    # "Si SET Z manual"
                    n134 = global write "cRIO_ZNB_AMI_GLOBALES.vi" "Target Z(T)"("Target Z(T)") -> ()
                    n135 = global write "cRIO_ZNB_AMI_GLOBALES.vi" "Rate Z(T/min)"("Rate Z(T/min)") -> ()
                    n136 = Bundle By Name(cluster=w267, "targetField"="Target Z(T)", "rampRate"="Rate Z(T/min)") -> (w254:T3)
                    n137 = local write "Settings Z"(w254) -> ()
                    n138 = call "AMI 430_Hardware_Module_Z AXIS.vi"("Enable"=TRUE, "Command"=AMI_430_Hardware_Module."SET  RAMPA", "error in (no error)"=w257, "Settings"=w254, "Comm Config In"=w255) -> ("error out"=w263:errorcluster)  [unwired: 2 in, 4 out]
                    n139 = call "Time Delay9"("error in (no error)"=w263, "Delay Time (s)"=w253) -> ("error out"=w262:errorcluster)  [unwired: 9 in]
                    n140 = global write "cRIO_ZNB_AMI_GLOBALES.vi" "Remote SET Z"(FALSE ("Remote SET X")) -> ()
                    n141 = local write "Remote SET Z"(FALSE ("Remote SET X")) -> ()
                    n142 = local write "SET Z"(FALSE ("Remote SET X")) -> ()
                    n143 = call "AMI 430_Hardware_Module_Z AXIS.vi"("Enable"=TRUE, "Command"=AMI_430_Hardware_Module."SET CAMPO", "error in (no error)"=w262, "Settings"=w254, "Comm Config In"=w255) -> ("error out"=w256:errorcluster)  [unwired: 2 in, 4 out]
                  }
                }
                n144 = local write "String"("Cambio parámetros eje Z ..." ("String")) -> ()
              }
            }
          }
          frame 4 {
            n145 = global read "cRIO_ZNB_AMI_GLOBALES.vi" "Remote RAMP X"() -> (w273:bool)
            n146 = Or(x=w273, y="RAMP X") -> (x .or. y?=w272:bool)
            n147 = case shown="True" w272 {
              tunnel: w278 -> [_ w282]
              tunnel: w277 -> [w279 w286]
              tunnel: [w279 w285] -> w276
              tunnel: w274 -> [_ w284]
              tunnel: "RAMP X" -> [_ w283]
              tunnel: w271 -> [_ _]
              tunnel: w270 -> [_ _]
              tunnel: w268 -> [_ w281]
              frame False {
              }
              frame True {
                # "Si RAMP  X manual o remoto..."
                n148 = case shown="False" w283 {
                  tunnel: w286 -> [w290 w305]
                  tunnel: [w291 w304] -> w285
                  tunnel: w284 -> [w289 w303]
                  tunnel: w281 -> [w288 w300]
                  tunnel: w282 -> [w287 w301]
                  frame False {
                    # "Si RAMP X remoto"
                    n149 = global read "cRIO_ZNB_AMI_GLOBALES.vi" "rampingMode X"() -> (w296:u16)
                    n150 = Bundle By Name(cluster=w287, "rampingMode"=w296) -> (w294:T3)
                    n151 = local write "rampingMode X"(w296) -> ()
                    n152 = local write "Settings X"(w294) -> ()
                    n153 = call "AMI 430_Hardware_Module_X AXIS.vi"("Enable"=TRUE, "Command"=AMI_430_Hardware_Module."SET RAMPING MODE", "error in (no error)"=w290, "Settings"=w294, "Comm Config In"=w288) -> ("error out"=w295:errorcluster)  [unwired: 2 in, 4 out]
                    n154 = global write "cRIO_ZNB_AMI_GLOBALES.vi" "Remote RAMP X"(FALSE ("Remote SET X")) -> ()
                    n155 = local write "Remote RAMP X"(FALSE ("Remote SET X")) -> ()
                    n156 = local write "RAMP X"(FALSE ("Remote SET X")) -> ()
                    n157 = call "Time Delay11"("error in (no error)"=w295, "Delay Time (s)"=w289) -> ("error out"=w291:errorcluster)  [unwired: 9 in]
                  }
                  frame True {
                    # "Si RAMP X manual"
                    n158 = Bundle By Name(cluster=w301, "rampingMode"="rampingMode X") -> (w308:T3)
                    n159 = global write "cRIO_ZNB_AMI_GLOBALES.vi" "rampingMode X"("rampingMode X") -> ()
                    n160 = local write "Settings X"(w308) -> ()
                    n161 = call "AMI 430_Hardware_Module_X AXIS.vi"("Enable"=TRUE, "Command"=AMI_430_Hardware_Module."SET RAMPING MODE", "error in (no error)"=w305, "Settings"=w308, "Comm Config In"=w300) -> ("error out"=w309:errorcluster)  [unwired: 2 in, 4 out]
                    n162 = global write "cRIO_ZNB_AMI_GLOBALES.vi" "Remote RAMP X"(FALSE ("Remote SET X")) -> ()
                    n163 = local write "Remote RAMP X"(FALSE ("Remote SET X")) -> ()
                    n164 = local write "RAMP X"(FALSE ("Remote SET X")) -> ()
                    n165 = call "Time Delay6"("error in (no error)"=w309, "Delay Time (s)"=w303) -> ("error out"=w304:errorcluster)  [unwired: 9 in]
                  }
                }
                n166 = local write "String"("Cambio modo de rampa eje X ..." ("String")) -> ()
              }
            }
          }
          frame 5 {
            n167 = global read "cRIO_ZNB_AMI_GLOBALES.vi" "Remote RAMP Y"() -> (w318:bool)
            n168 = Or(x=w318, y="RAMP Y") -> (x .or. y?=w317:bool)
            n169 = case shown="True" w317 {
              tunnel: w323 -> [_ _]
              tunnel: w322 -> [w324 w331]
              tunnel: [w324 w330] -> w321
              tunnel: w319 -> [_ w329]
              tunnel: "RAMP Y" -> [_ w328]
              tunnel: w316 -> [_ _]
              tunnel: w315 -> [_ w326]
              tunnel: w314 -> [_ w327]
              frame False {
              }
              frame True {
                # "Si RAMP  Y manual o remoto..."
                n170 = case shown="True" w328 {
                  tunnel: w331 -> [w335 w350]
                  tunnel: [w336 w349] -> w330
                  tunnel: w329 -> [w334 w348]
                  tunnel: w327 -> [w333 w346]
                  tunnel: w326 -> [w332 w347]
                  frame False {
                    # "Si RAMP Y remoto"
                    n171 = global read "cRIO_ZNB_AMI_GLOBALES.vi" "rampingMode Y"() -> (w341:u16)
                    n172 = Bundle By Name(cluster=w332, "rampingMode"=w341) -> (w339:T3)
                    n173 = local write "rampingMode Y"(w341) -> ()
                    n174 = local write "Settings Y"(w339) -> ()
                    n175 = call "AMI 430_Hardware_Module_Y AXIS.vi"("Enable"=TRUE, "Command"=AMI_430_Hardware_Module."SET RAMPING MODE", "error in (no error)"=w335, "Settings"=w339, "Comm Config In"=w333) -> ("error out"=w340:errorcluster)  [unwired: 2 in, 4 out]
                    n176 = global write "cRIO_ZNB_AMI_GLOBALES.vi" "Remote RAMP Y"(FALSE ("Remote SET X")) -> ()
                    n177 = local write "Remote RAMP Y"(FALSE ("Remote SET X")) -> ()
                    n178 = local write "RAMP Y"(FALSE ("Remote SET X")) -> ()
                    n179 = call "Time Delay16"("error in (no error)"=w340, "Delay Time (s)"=w334) -> ("error out"=w336:errorcluster)  [unwired: 9 in]
                  }
                  frame True {
                    # "Si RAMP Y manual"
                    n180 = Bundle By Name(cluster=w347, "rampingMode"="rampingMode Y") -> (w353:T3)
                    n181 = global write "cRIO_ZNB_AMI_GLOBALES.vi" "rampingMode Y"("rampingMode Y") -> ()
                    n182 = local write "Settings Y"(w353) -> ()
                    n183 = call "AMI 430_Hardware_Module_Y AXIS.vi"("Enable"=TRUE, "Command"=AMI_430_Hardware_Module."SET RAMPING MODE", "error in (no error)"=w350, "Settings"=w353, "Comm Config In"=w346) -> ("error out"=w354:errorcluster)  [unwired: 2 in, 4 out]
                    n184 = global write "cRIO_ZNB_AMI_GLOBALES.vi" "Remote RAMP Y"(FALSE ("Remote SET X")) -> ()
                    n185 = local write "Remote RAMP Y"(FALSE ("Remote SET X")) -> ()
                    n186 = local write "RAMP Y"(FALSE ("Remote SET X")) -> ()
                    n187 = call "Time Delay17"("error in (no error)"=w354, "Delay Time (s)"=w348) -> ("error out"=w349:errorcluster)  [unwired: 9 in]
                  }
                }
                n188 = local write "String"("Cambio modo de rampa eje Y ..." ("String")) -> ()
              }
            }
          }
          frame 6 {
            n189 = global read "cRIO_ZNB_AMI_GLOBALES.vi" "Remote RAMP Z"() -> (w363:bool)
            n190 = Or(x=w363, y="RAMP Z") -> (x .or. y?=w362:bool)
            n191 = case shown="True" w362 {
              tunnel: w368 -> [_ _]
              tunnel: w367 -> [w369 w376]
              tunnel: [w369 w375] -> w366
              tunnel: w364 -> [_ w374]
              tunnel: "RAMP Z" -> [_ w373]
              tunnel: w361 -> [_ w371]
              tunnel: w360 -> [_ _]
              tunnel: w358 -> [_ w372]
              frame False {
              }
              frame True {
                # "Si RAMP  Z manual o remoto..."
                n192 = case shown="False" w373 {
                  tunnel: w376 -> [w380 w395]
                  tunnel: [w381 w394] -> w375
                  tunnel: w374 -> [w379 w393]
                  tunnel: w372 -> [w378 w391]
                  tunnel: w371 -> [w377 w392]
                  frame False {
                    # "Si RAMP X remoto"
                    n193 = global read "cRIO_ZNB_AMI_GLOBALES.vi" "rampingMode Z"() -> (w386:u16)
                    n194 = Bundle By Name(cluster=w377, "rampingMode"=w386) -> (w384:T3)
                    n195 = local write "rampingMode Z"(w386) -> ()
                    n196 = local write "Settings Z"(w384) -> ()
                    n197 = call "AMI 430_Hardware_Module_Z AXIS.vi"("Enable"=TRUE, "Command"=AMI_430_Hardware_Module."SET RAMPING MODE", "error in (no error)"=w380, "Settings"=w384, "Comm Config In"=w378) -> ("error out"=w385:errorcluster)  [unwired: 2 in, 4 out]
                    n198 = global write "cRIO_ZNB_AMI_GLOBALES.vi" "Remote RAMP Z"(FALSE ("Remote SET X")) -> ()
                    n199 = local write "Remote RAMP Z"(FALSE ("Remote SET X")) -> ()
                    n200 = local write "RAMP Z"(FALSE ("Remote SET X")) -> ()
                    n201 = call "Time Delay19"("error in (no error)"=w385, "Delay Time (s)"=w379) -> ("error out"=w381:errorcluster)  [unwired: 9 in]
                  }
                  frame True {
                    # "Si RAMP Z manual"
                    n202 = global write "cRIO_ZNB_AMI_GLOBALES.vi" "rampingMode Z"("rampingMode Z") -> ()
                    n203 = Bundle By Name(cluster=w392, "rampingMode"="rampingMode Z") -> (w398:T3)
                    n204 = local write "Settings Z"(w398) -> ()
                    n205 = call "AMI 430_Hardware_Module_Z AXIS.vi"("Enable"=TRUE, "Command"=AMI_430_Hardware_Module."SET RAMPING MODE", "error in (no error)"=w395, "Settings"=w398, "Comm Config In"=w391) -> ("error out"=w399:errorcluster)  [unwired: 2 in, 4 out]
                    n206 = global write "cRIO_ZNB_AMI_GLOBALES.vi" "Remote RAMP Z"(FALSE ("Remote SET X")) -> ()
                    n207 = local write "Remote RAMP Z"(FALSE ("Remote SET X")) -> ()
                    n208 = local write "RAMP Z"(FALSE ("Remote SET X")) -> ()
                    n209 = call "Time Delay20"("error in (no error)"=w399, "Delay Time (s)"=w393) -> ("error out"=w394:errorcluster)  [unwired: 9 in]
                  }
                }
                n210 = local write "String"("Cambio modo de rampa eje Z ..." ("String")) -> ()
              }
            }
          }
          frame 7 {
            n211 = global read "cRIO_ZNB_AMI_GLOBALES.vi" "remoteVector"() -> (w408:bool)
            n212 = Or(x=w408, y="Vector") -> (x .or. y?=w407:bool)
            n213 = case shown="True" w407 {
              tunnel: w413 -> [_ _]
              tunnel: w412 -> [w414 w421]
              tunnel: [w414 w420] -> w411
              tunnel: w409 -> [_ w419]
              tunnel: "Vector" -> [_ w418]
              tunnel: w406 -> [_ w416]
              tunnel: w405 -> [_ _]
              tunnel: w404 -> [_ w417]
              frame False {
              }
              frame True {
                # "Si RAMP  Z manual o remoto..."
                n214 = case shown="False" w418 {
                  tunnel: w421 -> [w425 w440]
                  tunnel: [w426 w439] -> w420
                  tunnel: w419 -> [w424 w438]
                  tunnel: w417 -> [w423 w436]
                  tunnel: w416 -> [w422 w437]
                  frame False {
                    # "Si RAMP X remoto"
                    n215 = global read "cRIO_ZNB_AMI_GLOBALES.vi" "rampingMode Z"() -> (w431:u16)
                    n216 = Bundle By Name(cluster=w422, "rampingMode"=w431) -> (w429:T3)
                    n217 = local write "rampingMode Z 2"(w431) -> ()
                    n218 = local write "Settings Z"(w429) -> ()
                    n219 = call "AMI 430_Hardware_Module_Z AXIS.vi"("Enable"=TRUE, "Command"=AMI_430_Hardware_Module."SET RAMPING MODE", "error in (no error)"=w425, "Settings"=w429, "Comm Config In"=w423) -> ("error out"=w430:errorcluster)  [unwired: 2 in, 4 out]
                    n220 = global write "cRIO_ZNB_AMI_GLOBALES.vi" "Remote RAMP Z"(FALSE ("Remote SET X")) -> ()
                    n221 = local write "Remote RAMP Z"(FALSE ("Remote SET X")) -> ()
                    n222 = local write item#-1(FALSE ("Remote SET X")) -> ()
                    n223 = call "Time Delay8"("error in (no error)"=w430, "Delay Time (s)"=w424) -> ("error out"=w426:errorcluster)  [unwired: 9 in]
                  }
                  frame True {
                    # "Si RAMP Z manual"
                    n224 = global write "cRIO_ZNB_AMI_GLOBALES.vi" "rampingMode Z"("rampingMode Z 2") -> ()
                    n225 = Bundle By Name(cluster=w437, "rampingMode"="rampingMode Z 2") -> (w443:T3)
                    n226 = local write "Settings Z"(w443) -> ()
                    n227 = call "AMI 430_Hardware_Module_Z AXIS.vi"("Enable"=TRUE, "Command"=AMI_430_Hardware_Module."SET RAMPING MODE", "error in (no error)"=w440, "Settings"=w443, "Comm Config In"=w436) -> ("error out"=w444:errorcluster)  [unwired: 2 in, 4 out]
                    n228 = global write "cRIO_ZNB_AMI_GLOBALES.vi" "Remote RAMP Z"(FALSE ("Remote SET X")) -> ()
                    n229 = local write "Remote RAMP Z"(FALSE ("Remote SET X")) -> ()
                    n230 = local write item#-1(FALSE ("Remote SET X")) -> ()
                    n231 = call "Time Delay15"("error in (no error)"=w444, "Delay Time (s)"=w438) -> ("error out"=w439:errorcluster)  [unwired: 9 in]
                  }
                }
                n232 = local write "String"("Cambio parametros XYZ ..." ("String")) -> ()
              }
            }
          }
          frame 7 {
            n233 = global read "cRIO_ZNB_AMI_GLOBALES.vi" "Remote DEMAG X"() -> (w453:bool)
            n234 = Or(x=w453, y="Demag X") -> (x .or. y?=w452:bool)
            n235 = case shown="True" w452 {
              tunnel: w458 -> [_ w462]
              tunnel: w457 -> [w459 w466]
              tunnel: [w459 w465] -> w456
              tunnel: w454 -> [_ w464]
              tunnel: "Demag X" -> [_ w463]
              tunnel: w451 -> [_ _]
              tunnel: w450 -> [_ _]
              tunnel: w449 -> [_ w461]
              frame False {
              }
              frame True {
                # "Si DEMAG  X manual o remoto..."
                n236 = case shown="True" w463 {
                  tunnel: w466 -> [w467 w480]
                  tunnel: [w467 w484] -> w465
                  tunnel: w464 -> [_ w470]
                  tunnel: w461 -> [_ w478]
                  tunnel: w462 -> [_ w483]
                  frame False {
                    # "Si RAMP X remoto"
                  }
                  frame True {
                    w482 = u16 0 items=["RAMP", "PAUSE", "MANUAL UP", "MANUAL DOWN", "ZERO"] ("rampingMode X 2")
                    # "Si RAMP X manual"
                    n237 = call "AMI_Desimana X axis.vi"("error in (no error)"=w480) -> ("error out"=w479:errorcluster, "resulting string X"=w481:string)  [unwired: 7 in]
                    n238 = call "AMI_Parse_Desimanar_X.vi"("error in (no error)"=w479, "String"=w481) -> ("error out"=w475:errorcluster, "X Wait secs"=w469:dbl, "X Rate"=w473:dbl, "X Steps"=w474:i32)  [unwired: 6 in]
                    n239 = Bundle By Name(cluster=w483, "rampingMode"=w482) -> (w477:T3)
                    n240 = global write "cRIO_ZNB_AMI_GLOBALES.vi" "rampingMode X"(w482) -> ()
                    n241 = local write "rampingMode X"(w482) -> ()
                    n242 = global read "cRIO_ZNB_AMI_GLOBALES.vi" "X field (T)"() -> (w472:dbl)
                    n243 = call "Demag_fields.vi"("error in (no error)"=w475, "Steps"=w474, "Field (T)"=w472) -> ("error out"=w476:errorcluster, "Fields"=w471:dbl[])  [unwired: 7 in]
                    n244 = local write "Settings X"(w477) -> ()
                    n245 = for {
                      tunnel: w470 -> [w491]
                      tunnel: w478 -> [w496]
                      tunnel: w477 -> [w495]
                      shift-right: [w489] -> w484
                      shift-left: w476 -> [w493]
                      tunnel: w473 -> [w486]
                      tunnel: w471 -> [w485] mode=indexing
                      tunnel: w469 -> [w488]
                      tunnel: [FALSE ("Remote SET X")] -> w468
                      n246 = Bundle By Name(cluster=w495, "targetField"=w485, "rampRate"=w486) -> (w494:T3)
                      n247 = global write "cRIO_ZNB_AMI_GLOBALES.vi" "Rate X(T/min)"(w486) -> ()
                      n248 = local write "Rate X(T/min)"(w486) -> ()
                      n249 = global write "cRIO_ZNB_AMI_GLOBALES.vi" "Target X(T)"(w485) -> ()
                      n250 = local write "Target X(T)"(w485) -> ()
                      n251 = local write "Settings X"(w494) -> ()
                      n252 = call "AMI 430_Hardware_Module_X AXIS.vi"("Enable"=TRUE, "Command"=AMI_430_Hardware_Module."SET  RAMPA", "error in (no error)"=w493, "Settings"=w494, "Comm Config In"=w496) -> ("error out"=w503:errorcluster)  [unwired: 2 in, 4 out]
                      n253 = call "Time Delay7"("error in (no error)"=w503, "Delay Time (s)"=w491) -> ("error out"=w504:errorcluster)  [unwired: 9 in]
                      n254 = call "AMI 430_Hardware_Module_X AXIS.vi"("Enable"=TRUE, "Command"=AMI_430_Hardware_Module."SET CAMPO", "error in (no error)"=w504, "Settings"=w494, "Comm Config In"=w496) -> ("error out"=w498:errorcluster)  [unwired: 2 in, 4 out]
                      n255 = call "Time Delay12"("error in (no error)"=w498, "Delay Time (s)"=w491) -> ("error out"=w497:errorcluster)  [unwired: 9 in]
                      n256 = call "AMI 430_Hardware_Module_X AXIS.vi"("Enable"=TRUE, "Command"=AMI_430_Hardware_Module."SET RAMPING MODE", "error in (no error)"=w497, "Settings"=w494, "Comm Config In"=w496) -> ("error out"=w507:errorcluster)  [unwired: 2 in, 4 out]
                      n257 = call "Time Delay10"("error in (no error)"=w507, "Delay Time (s)"=w491) -> ("error out"=w492:errorcluster)  [unwired: 9 in]
                      n258 = while {
                        shift-right: [w512] -> w490
                        shift-left: w492 -> [w514]
                        tunnel: w491 -> [w511]
                        stop <- w509 stop-if-true
                        w517 = T2 1 items=["Unknown", "RAMPING to target field/current", "HOLDING at the target field/current", "PAUSED", "Ramping in MANUAL UP mode", "Ramping in MANUAL DOWN mode", "ZEROING CURRENT (in progress)", "Quench detected", "At ZERO current", "Heating persistent switch", "Cooling persistent switch", "External Rampdown active"] ("y")
                        n259 = property on="Refresh" class="Bool (strict)"(error in=w514, "Value"=TRUE ("Refresh")) -> (error out=w519:errorcluster)  [unwired: 1 in, 1 out]
                        n260 = call "AMI 430_Hardware_Module_X AXIS.vi"("Enable"=TRUE, "Command"=AMI_430_Hardware_Module."READ CAMPO", "error in (no error)"=w519) -> ("error out"=w526:errorcluster, "magneticField"=w529:dbl)  [unwired: 4 in, 3 out]
                        n261 = call "AMI 430_Hardware_Module_X AXIS.vi"("Enable"=TRUE, "Command"=AMI_430_Hardware_Module."STATUS", "error in (no error)"=w526) -> ("error out"=w518:errorcluster, "state"=w516:T2)  [unwired: 4 in, 3 out]
                        n262 = global read "cRIO_ZNB_AMI_GLOBALES.vi" "Z field (T)"() -> (w527:dbl)
                        n263 = global read "cRIO_ZNB_AMI_GLOBALES.vi" "Y field (T)"() -> (w528:dbl)
                        n264 = global write "cRIO_ZNB_AMI_GLOBALES.vi" "X field (T)"(w529) -> ()
                        n265 = local write "X field (T)"(w529) -> ()
                        n266 = global write "cRIO_ZNB_AMI_GLOBALES.vi" "X state"(w516) -> ()
                        n267 = local write "X state"(w516) -> ()
                        n268 = property on="Refresh" class="Bool (strict)"(error in=w518, "Value"=FALSE ("Refresh")) -> (error out=w513:errorcluster)  [unwired: 1 in, 1 out]
                        n269 = Equal?(x=w516, y=w517) -> (x = y?=w515:bool)
                        n270 = Bundle("Z field (T)"=w527, "Y field (T)"=w528, "magneticField"=w529) -> (w530:T8)  [unwired: 1 in]
                        n271 = local write "X ramping"(w515) -> ()
                        n272 = global write "cRIO_ZNB_AMI_GLOBALES.vi" "X ramping"(w515) -> ()
                        n273 = local write "Waveform Chart"(w530) -> ()
                        n274 = call "Time Delay13"("error in (no error)"=w513, "Delay Time (s)"=w511) -> ("error out"=w512:errorcluster)  [unwired: 9 in]
                        n275 = Not(x=w515) -> (.not. x?=w510:bool)
                        n276 = Or(x=w510, y=FALSE ("Refresh")) -> (x .or. y?=w509:bool)
                      }
                      n277 = call "Time Delay14"("error in (no error)"=w490, "Delay Time (s)"=w488) -> ("error out"=w489:errorcluster)  [unwired: 9 in]
                    }
                    n278 = global write "cRIO_ZNB_AMI_GLOBALES.vi" "Remote DEMAG X"(w468) -> ()
                    n279 = local write "Remote DEMAG X"(w468) -> ()
                    n280 = local write "Demag X"(w468) -> ()
                  }
                }
                n281 = local write "String"("Desmagnetizando eje X ... ESPERE..." ("String")) -> ()
              }
            }
          }
          frame 8 {
            n282 = global read "cRIO_ZNB_AMI_GLOBALES.vi" "Remote DEMAG Y"() -> (w536:bool)
            n283 = Or(x=w536, y="Demag Y") -> (x .or. y?=w535:bool)
            n284 = case shown="True" w535 {
              tunnel: w541 -> [_ w546]
              tunnel: w540 -> [w542 w550]
              tunnel: [w542 w549] -> w539
              tunnel: w537 -> [_ w548]
              tunnel: "Demag Y" -> [_ w547]
              tunnel: w534 -> [_ _]
              tunnel: w533 -> [_ w543]
              tunnel: w531 -> [_ w545]
              frame False {
              }
              frame True {
                # "Si DEMAG  Y manual o remoto..."
                n285 = case shown="True" w547 {
                  tunnel: w550 -> [w551 w565]
                  tunnel: [w551 w568] -> w549
                  tunnel: w548 -> [_ w555]
                  tunnel: w545 -> [_ w563]
                  tunnel: w546 -> [_ _]
                  tunnel: w543 -> [_ w552]
                  frame False {
                    # "Si RAMP Y remoto"
                  }
                  frame True {
                    w567 = u16 0 items=["RAMP", "PAUSE", "MANUAL UP", "MANUAL DOWN", "ZERO"] ("rampingMode X 2")
                    # "Si RAMP Y manual"
                    n286 = call "AMI_Desimana Y axis.vi"("error in (no error)"=w565) -> ("error out"=w564:errorcluster, "resulting string Y"=w566:string)  [unwired: 7 in]
                    n287 = call "AMI_Parse_Desimanar_Y.vi"("error in (no error)"=w564, "String"=w566) -> ("error out"=w560:errorcluster, "Y Wait secs"=w554:i32, "Y Rate"=w558:dbl, "Y Steps"=w559:i32)  [unwired: 6 in]
                    n288 = Bundle By Name(cluster=w552, "rampingMode"=w567) -> (w562:T3)
                    n289 = global write "cRIO_ZNB_AMI_GLOBALES.vi" "rampingMode Y"(w567) -> ()
                    n290 = local write "rampingMode Y"(w567) -> ()
                    n291 = global read "cRIO_ZNB_AMI_GLOBALES.vi" "Y field (T)"() -> (w557:dbl)
                    n292 = call "Demag_fields.vi"("error in (no error)"=w560, "Steps"=w559, "Field (T)"=w557) -> ("error out"=w561:errorcluster, "Fields"=w556:dbl[])  [unwired: 7 in]
                    n293 = local write "Settings Y"(w562) -> ()
                    n294 = for {
                      tunnel: w555 -> [w575]
                      tunnel: w563 -> [w580]
                      tunnel: w562 -> [w579]
                      shift-right: [w573] -> w568
                      shift-left: w561 -> [w577]
                      tunnel: w558 -> [w570]
                      tunnel: w556 -> [w569] mode=indexing
                      tunnel: w554 -> [w572]
                      tunnel: [FALSE ("Remote SET X")] -> w553
                      n295 = Bundle By Name(cluster=w579, "targetField"=w569, "rampRate"=w570) -> (w578:T3)
                      n296 = global write "cRIO_ZNB_AMI_GLOBALES.vi" "Rate Y(T/min)"(w570) -> ()
                      n297 = local write "Rate Y(T/min)"(w570) -> ()
                      n298 = global write "cRIO_ZNB_AMI_GLOBALES.vi" "Target Y(T)"(w569) -> ()
                      n299 = local write "Target Y(T)"(w569) -> ()
                      n300 = local write "Settings Y"(w578) -> ()
                      n301 = call "AMI 430_Hardware_Module_Y AXIS.vi"("Enable"=TRUE, "Command"=AMI_430_Hardware_Module."SET  RAMPA", "error in (no error)"=w577, "Settings"=w578, "Comm Config In"=w580) -> ("error out"=w587:errorcluster)  [unwired: 2 in, 4 out]
                      n302 = call "Time Delay21"("error in (no error)"=w587, "Delay Time (s)"=w575) -> ("error out"=w588:errorcluster)  [unwired: 9 in]
                      n303 = call "AMI 430_Hardware_Module_Y AXIS.vi"("Enable"=TRUE, "Command"=AMI_430_Hardware_Module."SET CAMPO", "error in (no error)"=w588, "Settings"=w578, "Comm Config In"=w580) -> ("error out"=w582:errorcluster)  [unwired: 2 in, 4 out]
                      n304 = call "Time Delay22"("error in (no error)"=w582, "Delay Time (s)"=w575) -> ("error out"=w581:errorcluster)  [unwired: 9 in]
                      n305 = call "AMI 430_Hardware_Module_Y AXIS.vi"("Enable"=TRUE, "Command"=AMI_430_Hardware_Module."SET RAMPING MODE", "error in (no error)"=w581, "Settings"=w578, "Comm Config In"=w580) -> ("error out"=w591:errorcluster)  [unwired: 2 in, 4 out]
                      n306 = call "Time Delay18"("error in (no error)"=w591, "Delay Time (s)"=w575) -> ("error out"=w576:errorcluster)  [unwired: 9 in]
                      n307 = while {
                        shift-right: [w598] -> w574
                        shift-left: w576 -> [w600]
                        tunnel: w575 -> [w597]
                        stop <- w595 stop-if-true
                        w603 = T2 1 items=["Unknown", "RAMPING to target field/current", "HOLDING at the target field/current", "PAUSED", "Ramping in MANUAL UP mode", "Ramping in MANUAL DOWN mode", "ZEROING CURRENT (in progress)", "Quench detected", "At ZERO current", "Heating persistent switch", "Cooling persistent switch", "External Rampdown active"] ("y")
                        n308 = property on="Refresh" class="Bool (strict)"(error in=w600, "Value"=TRUE ("Refresh")) -> (error out=w605:errorcluster)  [unwired: 1 in, 1 out]
                        n309 = call "AMI 430_Hardware_Module_Y AXIS.vi"("Enable"=TRUE, "Command"=AMI_430_Hardware_Module."READ CAMPO", "error in (no error)"=w605) -> ("error out"=w612:errorcluster, "magneticField"=w592:dbl)  [unwired: 4 in, 3 out]
                        n310 = call "AMI 430_Hardware_Module_Y AXIS.vi"("Enable"=TRUE, "Command"=AMI_430_Hardware_Module."STATUS", "error in (no error)"=w612) -> ("error out"=w604:errorcluster, "state"=w602:T2)  [unwired: 4 in, 3 out]
                        n311 = global read "cRIO_ZNB_AMI_GLOBALES.vi" "Z field (T)"() -> (w613:dbl)
                        n312 = global write "cRIO_ZNB_AMI_GLOBALES.vi" "Y field (T)"(w592) -> ()
                        n313 = global read "cRIO_ZNB_AMI_GLOBALES.vi" "X field (T)"() -> (w593:dbl)
                        n314 = local write "Y field (T)"(w592) -> ()
                        n315 = global write "cRIO_ZNB_AMI_GLOBALES.vi" "Y state"(w602) -> ()
                        n316 = local write "Y state"(w602) -> ()
                        n317 = property on="Refresh" class="Bool (strict)"(error in=w604, "Value"=FALSE ("Refresh")) -> (error out=w599:errorcluster)  [unwired: 1 in, 1 out]
                        n318 = Equal?(x=w602, y=w603) -> (x = y?=w601:bool)
                        n319 = Bundle("Z field (T)"=w613, "magneticField"=w592, "X field (T)"=w593) -> (w614:T9)  [unwired: 1 in]
                        n320 = local write "Y ramping"(w601) -> ()
                        n321 = global write "cRIO_ZNB_AMI_GLOBALES.vi" "Y ramping"(w601) -> ()
                        n322 = local write "Waveform Chart"(w614) -> ()
                        n323 = call "Time Delay23"("error in (no error)"=w599, "Delay Time (s)"=w597) -> ("error out"=w598:errorcluster)  [unwired: 9 in]
                        n324 = Not(x=w601) -> (.not. x?=w596:bool)
                        n325 = Or(x=w596, y=FALSE ("Refresh")) -> (x .or. y?=w595:bool)
                      }
                      n326 = call "Time Delay24"("error in (no error)"=w574, "Delay Time (s)"=w572) -> ("error out"=w573:errorcluster)  [unwired: 9 in]
                    }
                    n327 = global write "cRIO_ZNB_AMI_GLOBALES.vi" "Remote DEMAG Y"(w553) -> ()
                    n328 = local write "Remote DEMAG Y"(w553) -> ()
                    n329 = local write "Demag Y"(w553) -> ()
                  }
                }
                n330 = local write "String"("Desmagnetizando eje Y ... ESPERE..." ("String")) -> ()
              }
            }
          }
          frame 9 {
            n331 = global read "cRIO_ZNB_AMI_GLOBALES.vi" "Remote DEMAG Z"() -> (w620:bool)
            n332 = Or(x=w620, y="Demag Z") -> (x .or. y?=w619:bool)
            n333 = case shown="True" w619 {
              tunnel: w625 -> [_ _]
              tunnel: w624 -> [w626 w633]
              tunnel: [w626 w632] -> w623
              tunnel: w621 -> [_ w631]
              tunnel: "Demag Z" -> [_ w630]
              tunnel: w618 -> [_ w627]
              tunnel: w617 -> [_ _]
              tunnel: w615 -> [_ w629]
              frame False {
              }
              frame True {
                # "Si DEMAG  Z manual o remoto..."
                n334 = case shown="True" w630 {
                  tunnel: w633 -> [w634 w648]
                  tunnel: [w634 w651] -> w632
                  tunnel: w631 -> [_ w638]
                  tunnel: w629 -> [_ w646]
                  tunnel: w627 -> [_ w635]
                  frame False {
                    # "Si RAMP Z remoto"
                  }
                  frame True {
                    w650 = u16 0 items=["RAMP", "PAUSE", "MANUAL UP", "MANUAL DOWN", "ZERO"] ("rampingMode X 2")
                    # "Si RAMP Z manual"
                    n335 = call "AMI_Desimana Z axis.vi"("error in (no error)"=w648) -> ("error out"=w647:errorcluster, "resulting string Z"=w649:string)  [unwired: 7 in]
                    n336 = call "AMI_Parse_Desimanar_Z.vi"("error in (no error)"=w647, "String"=w649) -> ("error out"=w643:errorcluster, "Z Wait secs"=w637:i32, "Z Rate"=w641:dbl, "Z Steps"=w642:i32)  [unwired: 6 in]
                    n337 = Bundle By Name(cluster=w635, "rampingMode"=w650) -> (w645:T3)
                    n338 = global write "cRIO_ZNB_AMI_GLOBALES.vi" "rampingMode Z"(w650) -> ()
                    n339 = local write "rampingMode Z"(w650) -> ()
                    n340 = global read "cRIO_ZNB_AMI_GLOBALES.vi" "Z field (T)"() -> (w640:dbl)
                    n341 = call "Demag_fields.vi"("error in (no error)"=w643, "Steps"=w642, "Field (T)"=w640) -> ("error out"=w644:errorcluster, "Fields"=w639:dbl[])  [unwired: 7 in]
                    n342 = local write "Settings Z"(w645) -> ()
                    n343 = for {
                      tunnel: w638 -> [w658]
                      tunnel: w646 -> [w663]
                      tunnel: w645 -> [w662]
                      shift-right: [w656] -> w651
                      shift-left: w644 -> [w660]
                      tunnel: w641 -> [w653]
                      tunnel: w639 -> [w652] mode=indexing
                      tunnel: w637 -> [w655]
                      tunnel: [FALSE ("Remote SET X")] -> w636
                      n344 = Bundle By Name(cluster=w662, "targetField"=w652, "rampRate"=w653) -> (w661:T3)
                      n345 = global write "cRIO_ZNB_AMI_GLOBALES.vi" "Rate Z(T/min)"(w653) -> ()
                      n346 = local write "Rate Z(T/min)"(w653) -> ()
                      n347 = global write "cRIO_ZNB_AMI_GLOBALES.vi" "Target Z(T)"(w652) -> ()
                      n348 = local write "Target Z(T)"(w652) -> ()
                      n349 = local write "Settings Z"(w661) -> ()
                      n350 = call "AMI 430_Hardware_Module_Z AXIS.vi"("Enable"=TRUE, "Command"=AMI_430_Hardware_Module."SET  RAMPA", "error in (no error)"=w660, "Settings"=w661, "Comm Config In"=w663) -> ("error out"=w670:errorcluster)  [unwired: 2 in, 4 out]
                      n351 = call "Time Delay27"("error in (no error)"=w670, "Delay Time (s)"=w658) -> ("error out"=w671:errorcluster)  [unwired: 9 in]
                      n352 = call "AMI 430_Hardware_Module_Z AXIS.vi"("Enable"=TRUE, "Command"=AMI_430_Hardware_Module."SET CAMPO", "error in (no error)"=w671, "Settings"=w661, "Comm Config In"=w663) -> ("error out"=w665:errorcluster)  [unwired: 2 in, 4 out]
                      n353 = call "Time Delay28"("error in (no error)"=w665, "Delay Time (s)"=w658) -> ("error out"=w664:errorcluster)  [unwired: 9 in]
                      n354 = call "AMI 430_Hardware_Module_Z AXIS.vi"("Enable"=TRUE, "Command"=AMI_430_Hardware_Module."SET RAMPING MODE", "error in (no error)"=w664, "Settings"=w661, "Comm Config In"=w663) -> ("error out"=w674:errorcluster)  [unwired: 2 in, 4 out]
                      n355 = call "Time Delay26"("error in (no error)"=w674, "Delay Time (s)"=w658) -> ("error out"=w659:errorcluster)  [unwired: 9 in]
                      n356 = while {
                        shift-right: [w681] -> w657
                        shift-left: w659 -> [w683]
                        tunnel: w658 -> [w680]
                        stop <- w678 stop-if-true
                        w686 = T2 1 items=["Unknown", "RAMPING to target field/current", "HOLDING at the target field/current", "PAUSED", "Ramping in MANUAL UP mode", "Ramping in MANUAL DOWN mode", "ZEROING CURRENT (in progress)", "Quench detected", "At ZERO current", "Heating persistent switch", "Cooling persistent switch", "External Rampdown active"] ("y")
                        n357 = property on="Refresh" class="Bool (strict)"(error in=w683, "Value"=TRUE ("Refresh")) -> (error out=w688:errorcluster)  [unwired: 1 in, 1 out]
                        n358 = call "AMI 430_Hardware_Module_Z AXIS.vi"("Enable"=TRUE, "Command"=AMI_430_Hardware_Module."READ CAMPO", "error in (no error)"=w688) -> ("error out"=w695:errorcluster, "magneticField"=w676:dbl)  [unwired: 4 in, 3 out]
                        n359 = call "AMI 430_Hardware_Module_Z AXIS.vi"("Enable"=TRUE, "Command"=AMI_430_Hardware_Module."STATUS", "error in (no error)"=w695) -> ("error out"=w687:errorcluster, "state"=w685:T2)  [unwired: 4 in, 3 out]
                        n360 = global write "cRIO_ZNB_AMI_GLOBALES.vi" "Z field (T)"(w676) -> ()
                        n361 = global read "cRIO_ZNB_AMI_GLOBALES.vi" "Y field (T)"() -> (w696:dbl)
                        n362 = global read "cRIO_ZNB_AMI_GLOBALES.vi" "X field (T)"() -> (w675:dbl)
                        n363 = local write "Z field (T)"(w676) -> ()
                        n364 = global write "cRIO_ZNB_AMI_GLOBALES.vi" "Z state"(w685) -> ()
                        n365 = local write "Z state"(w685) -> ()
                        n366 = property on="Refresh" class="Bool (strict)"(error in=w687, "Value"=FALSE ("Refresh")) -> (error out=w682:errorcluster)  [unwired: 1 in, 1 out]
                        n367 = Equal?(x=w685, y=w686) -> (x = y?=w684:bool)
                        n368 = Bundle("magneticField"=w676, "Y field (T)"=w696, "X field (T)"=w675) -> (w697:T10)  [unwired: 1 in]
                        n369 = local write "Z ramping"(w684) -> ()
                        n370 = global write "cRIO_ZNB_AMI_GLOBALES.vi" "Z ramping"(w684) -> ()
                        n371 = local write "Waveform Chart"(w697) -> ()
                        n372 = call "Time Delay29"("error in (no error)"=w682, "Delay Time (s)"=w680) -> ("error out"=w681:errorcluster)  [unwired: 9 in]
                        n373 = Not(x=w684) -> (.not. x?=w679:bool)
                        n374 = Or(x=w679, y=FALSE ("Refresh")) -> (x .or. y?=w678:bool)
                      }
                      n375 = call "Time Delay30"("error in (no error)"=w657, "Delay Time (s)"=w655) -> ("error out"=w656:errorcluster)  [unwired: 9 in]
                    }
                    n376 = global write "cRIO_ZNB_AMI_GLOBALES.vi" "Remote DEMAG Z"(w636) -> ()
                    n377 = local write "Remote DEMAG Z"(w636) -> ()
                    n378 = local write "Demag Z"(w636) -> ()
                  }
                }
                n379 = local write "String"("Desmagnetizando eje Z ... ESPERE..." ("String")) -> ()
              }
            }
          }
        }
        "Command" <- w54
        n380 = global read "cRIO_ZNB_AMI_GLOBALES.vi" "stopMagneticField"() -> (w67:bool)
        n381 = Unbundle By Name(w62) -> ("status"=→"ERROR":bool)
        n382 = call <vilib>:"Clear Errors.vi"("error in (no error)"=w62) -> ("error out"=w65:errorcluster)  [unwired: 5 in, 1 out]
        n383 = control-ref of="This VI"() -> (w68:refnum<vi>)
        n384 = Or(x="stop", y=w67) -> (x .or. y?=w72:bool)
        "Ciclo" <- w64
      }
      "Error Out" <- w50
      n385 = global write "cRIO_ZNB_AMI_GLOBALES.vi" "stopMagneticField"(w51) -> ()
      n386 = invoke class="VI" method="FP.Close"(reference=w52) -> ()  [unwired: 2 in, 3 out]
      "Remote SET Y" <- w11
      "Remote RAMP X" <- w14
      "Remote SET X" <- w13
      "Remote RAMP Z" <- w16
      "Remote SET Z" <- w12
      "Remote RAMP Y" <- w15
      "Remote DEMAG Y" <- w7
      "Remote DEMAG X" <- w6
      "Remote DEMAG Z" <- w5
    }
  }
  "String" <- w1
